vi "image_analysis_bkgndmagnetictrap.vi"(0 "2D Array In":i32[][](array[numeric]), 1 "File Path for \nbackground image":path=path "C:/data/MOT/08.05.02/metapictemp600c1v40a35msh100usd1.000motp0back.bmp", 2 "Ions or Neutral Atoms?":bool=TRUE, 3 "Delta_x (m)":dbl=2.33e-05 format="%.2e", 4 "Delta_y (m)":dbl=4.63e-05 format="%.2e", 5 "camera background with no image beam\nIt will be subtracted before the log is taken":i8=15, 6 "coilcurrent":dbl=40.0 format="%.2f", 7 "take new\nnew image":bool=TRUE, 8 "ROI Controls":T1, 10 "Image beam \nDetuning (MHz)":dbl=12.5 format="%.2f", 11 "Cut image?":bool, 12 "timeout(min 100ms)":u32=1000) -> (9 "Intensity Graph \natoms":sgl[][](graph), 13 "Intensity Graph \nbackground":sgl[][](graph), 14 "X  side":cluster{cluster{dbl, dbl}[]}[](graph)=[{[{0.0, -0.00023040071411132814}, {2.33e-05, -0.00023119197387695312}, {4.66e-05, -0.0002076152587890625}, {6.99e-05, -0.00020104497680664061}, {9.32e-05, -0.000178349951171875}, {0.0001165, -0.00020604686889648437}, {0.0001398, -0.00019964896850585938}, {0.0001631, -0.0001973317077636719}, {0.0001864, -0.00018958018798828126}, {0.0002097, -0.00018725162353515625}, {0.000233, -0.00018564649658203125}, {0.0002563, -0.0001972638854980469}, {0.0002796, -0.00018755399780273437}, {0.0003029, -0.00017615420532226563}, {0.0003262, -0.00017684373168945313}, {0.0003495, -0.00017816343994140626}, {0.0003728, -0.00018060221557617188}, {0.00039610000000000003, -0.00018643775634765626}, {0.0004194, -0.00021354122924804688}, {0.0004427, -0.00018863067626953125}, {0.000466, -0.00018703402709960938}, {0.0004893, -0.00018847242431640625}, {0.0005126, -0.00015889909057617189}, {0.0005359, -0.0001712625244140625}, {0.0005592, -0.00017300894775390625}, {0.0005825, -0.00016774424438476562}, {0.0006058, -0.00018329815063476563}, {0.0006291000000000001, -0.00014636327514648437}, {0.0006524, -0.00013831785888671874}, {0.0006757, -0.00016184935913085937}, {0.000699, -0.000178485595703125}, {0.0007223, -0.0001590545166015625}, {0.0007456, -0.00015677681884765626}, {0.0007689, -0.00013077545776367188}, {0.0007922000000000001, -0.00016876723022460937}, {0.0008155, -0.000126985888671875}, {0.0008388, -0.00016878983764648437}, {0.0008621, -0.00014658369750976562}, {0.0008854, -0.00016071333618164062}, {0.0009087, -0.00014554093017578125}, {0.000932, -0.00013422308959960938}, {0.0009553000000000001, -0.0001502178405761719}, {0.0009786, -0.00015147537841796876}, {0.0010019, -0.00014486270751953124}, {0.0010252, -0.00015495974731445314}, {0.0010485, -0.00012384345703125}, {0.0010718, -0.00012299850463867186}, {0.0010951000000000001, -0.00013838568115234374}, {0.0011184, -0.00016345731201171875}, {0.0011417, -0.0001566948669433594}, {0.001165, -0.00014931636962890626}, {0.0011883, -0.00010717896118164062}, {0.0012116, -0.00010879256591796875}, {0.0012349, -0.0001059722900390625}, {0.0012582000000000001, -0.0001241938720703125}, {0.0012815, -0.00013572083129882812}, {0.0013048, -0.00012067559204101562}, {0.0013281, -0.00012900077514648437}, {0.0013514, -9.90544189453125e-05}, {0.0013747, -0.0001157160888671875}, {0.001398, -0.00011736077880859375}, {0.0014213000000000001, -8.70498779296875e-05}, {0.0014446, -0.000123526953125}, {0.0014679, -0.0001004560791015625}, {0.0014912, -5.974576416015625e-05}, {0.0015145, -7.730042724609375e-05}, {0.0015378, -9.181156616210937e-05}, {0.0015611, -0.0001171064453125}, {0.0015844000000000001, -7.690197143554687e-05}, {0.0016077, -7.38019287109375e-05}, {0.001631, -9.62510986328125e-05}, {0.0016543, -4.338646850585937e-05}, {0.0016776, -9.5878076171875e-05}, {0.0017009, -7.96346435546875e-05}, {0.0017242, -7.93181396484375e-05}, {0.0017475000000000001, -6.642060546875e-05}, {0.0017708, -5.844301147460938e-05}, {0.0017941, -2.755279541015625e-05}, {0.0018174, -2.5744201660156252e-05}, {0.0018407, -5.0640625e-05}, {0.001864, -4.254151611328125e-05}, {0.0018873, -3.9766455078125e-05}, {0.0019106000000000001, -1.7760955810546876e-05}, {0.0019339000000000001, -2.0016046142578124e-05}, {0.0019572, -1.730032958984375e-05}, {0.0019805, 4.25584716796875e-06}, {0.0020038, -1.5260009765625e-06}, {0.0020271, 1.6353643798828126e-05}, {0.0020504, 4.45931396484375e-06}, {0.0020737, 1.56782470703125e-05}, {0.002097, 1.87754638671875e-05}, {0.0021203, 6.5250671386718754e-06}, {0.0021436, -7.1778564453125e-07}, {0.0021669000000000002, 2.6719146728515625e-05}, {0.0021902000000000002, 4.67182373046875e-05}, {0.0022135, 4.4092950439453123e-05}, {0.0022368, 5.912688598632813e-05}, {0.0022601, 6.413160400390626e-05}, {0.0022834, 5.6900054931640624e-05}, {0.0023067, 6.803703613281251e-05}, {0.00233, 8.644512939453125e-05}, {0.0023533, 7.566138916015625e-05}, {0.0023766, 6.502459716796875e-05}, {0.0023999, 8.933887939453125e-05}, {0.0024232, 9.000579833984375e-05}, {0.0024465, 0.0001182481201171875}, {0.0024698, 0.0001048871337890625}, {0.0024931000000000003, 0.0001308856689453125}, {0.0025164000000000002, 0.00013674946899414062}, {0.0025397, 0.0001610552734375}, {0.002563, 0.00014260196533203126}, {0.0025863, 0.0001531341979980469}, {0.0026096, 0.0001802150634765625}, {0.0026329, 0.00019327367553710937}, {0.0026562, 0.00022464429931640624}, {0.0026795, 0.000221123193359375}, {0.0027028, 0.00019760864868164063}, {0.0027261, 0.00019808905639648439}, {0.0027494, 0.00023230821533203126}, {0.0027727, 0.0002467458801269531}, {0.002796, 0.00025002678222656253}, {0.0028193000000000003, 0.00026431184692382814}, {0.0028426000000000002, 0.0002459941833496094}, {0.0028659000000000002, 0.00026929395751953126}, {0.0028892, 0.0003082606750488281}, {0.0029125, 0.0002984066650390625}, {0.0029358, 0.00030499107666015626}, {0.0029591, 0.00033020400390625}, {0.0029824, 0.0003341263916015625}, {0.0030057, 0.00035323531494140626}, {0.003029, 0.00035600755004882814}, {0.0030523, 0.00037995446166992186}, {0.0030756, 0.0003714258117675781}, {0.0030989, 0.0003785414978027344}, {0.0031222, 0.00038694580688476563}, {0.0031455, 0.0004150440063476563}, {0.0031688000000000003, 0.0004460359558105469}, {0.0031921000000000002, 0.0004576816040039063}, {0.0032154, 0.0004373829650878906}, {0.0032387, 0.00044043496704101564}, {0.003262, 0.00046968614501953124}, {0.0032853, 0.00046797928466796876}, {0.0033086, 0.0005343603271484375}, {0.0033319, 0.000518049072265625}, {0.0033552, 0.0005307911804199219}, {0.0033785, 0.0005506433227539062}, {0.0034018, 0.0005478513061523437}, {0.0034251, 0.0005569762268066407}, {0.0034484, 0.0005951799438476562}, {0.0034717, 0.0006168124206542969}, {0.0034950000000000003, 0.0006063564880371094}, {0.0035183000000000002, 0.0006301931884765625}, {0.0035416, 0.0006353505065917969}, {0.0035649, 0.0006507065979003907}, {0.0035882, 0.0006587463623046875}, {0.0036115, 0.0007066260559082031}, {0.0036348, 0.0006745715576171876}, {0.0036581, 0.0007187690673828125}, {0.0036814, 0.0007195122863769531}, {0.0037047, 0.0007214169616699219}, {0.003728, 0.0007334469360351563}, {0.0037513, 0.0007567438842773438}, {0.0037746, 0.0007910478210449218}, {0.0037979, 0.0007963803466796875}, {0.0038212000000000003, 0.0007861307067871094}, {0.0038445000000000003, 0.0008184621459960937}, {0.0038678000000000002, 0.0008249674316406251}, {0.0038911, 0.0008380316955566406}, {0.0039144, 0.0008839106323242187}, {0.0039377, 0.0008829582946777343}, {0.003961, 0.0009055233276367187}, {0.0039843000000000005, 0.0009045681640625}, {0.0040076, 0.0009299393432617188}, {0.0040309000000000005, 0.0009854631713867188}, {0.0040542, 0.0009813542724609375}, {0.0040775, 0.0009880488952636718}, {0.0041008, 0.001000581884765625}, {0.0041241, 0.0010300223999023437}, {0.0041474, 0.001029171795654297}, {0.0041707, 0.0010493347900390625}, {0.004194, 0.0010845712829589845}, {0.0042173, 0.0010739486206054688}, {0.0042406, 0.001092376495361328}, {0.0042639, 0.0011004558227539062}, {0.0042872, 0.0011284014221191407}, {0.0043105, 0.0011756170227050782}, {0.0043338000000000005, 0.001184140020751953}, {0.0043571, 0.0011864940185546875}, {0.0043804000000000004, 0.0012101272521972655}, {0.0044037, 0.001194449005126953}, {0.004427, 0.0012500717407226563}, {0.0044503, 0.0012585269165039062}, {0.0044736, 0.0012805493713378907}, {0.0044969, 0.0012812869384765625}, {0.0045202, 0.0012850680297851562}, {0.0045435, 0.001292859112548828}, {0.0045668, 0.0013328488159179688}, {0.0045901, 0.0013298702880859374}, {0.0046134, 0.0013652791625976563}, {0.0046367, 0.001366519744873047}, {0.00466, 0.0013854901977539062}, {0.0046833000000000005, 0.0014075380859375}, {0.0047066, 0.0014307163452148438}, {0.0047299, 0.001454810205078125}, {0.0047532, 0.0014336440063476563}, {0.0047765, 0.0014266159240722655}, {0.0047998, 0.0014909622985839843}, {0.0048231, 0.0014609170349121094}, {0.0048464, 0.0015016838684082032}, {0.0048697, 0.0015183624938964844}, {0.004893, 0.0015467969787597657}, {0.0049163, 0.0015608559692382813}, {0.0049396, 0.0015447057922363281}, {0.0049629, 0.0015464098266601562}, {0.0049862000000000005, 0.0015989127380371094}, {0.0050095, 0.001574869744873047}, {0.0050328000000000005, 0.00164387607421875}, {0.0050561, 0.001618668798828125}, {0.0050794, 0.0016376618591308594}, {0.0051027, 0.0016571861938476562}, {0.005126, 0.0016686396789550781}, {0.0051493, 0.0017015108703613282}, {0.0051726, 0.0016855048156738282}, {0.0051959, 0.001690854296875}, {0.0052192, 0.0017352072326660157}, {0.0052425, 0.001697243719482422}, {0.0052658, 0.001747906951904297}, {0.0052891, 0.0017650772888183593}, {0.0053124, 0.001771729522705078}, {0.0053357000000000005, 0.0017894961303710937}, {0.005359, 0.00176170595703125}, {0.0053823000000000005, 0.0017409551696777343}, {0.0054056, 0.0017913838500976562}, {0.0054289, 0.0017596119445800781}, {0.0054522, 0.0018210221801757812}, {0.0054755, 0.001803001239013672}, {0.0054988, 0.0018012209045410157}, {0.0055221, 0.0017957386047363281}, {0.0055454, 0.0017480991149902345}, {0.0055687, 0.0017993049255371095}, {0.005592, 0.0017956142639160156}, {0.0056153, 0.0017572579467773437}, {0.0056386000000000006, 0.0017667954528808594}, {0.0056619, 0.0017284334838867188}, {0.0056852000000000005, 0.0017505181091308595}, {0.0057085, 0.0017459655395507814}, {0.0057318000000000004, 0.0017314883117675781}, {0.0057551, 0.0017498059753417968}, {0.0057784, 0.0016802429382324219}, {0.0058017, 0.0016734070190429688}, {0.005825, 0.0017002109436035156}, {0.0058483, 0.0016686877197265625}, {0.0058716, 0.0016841088073730468}, {0.0058949, 0.0016317697998046875}, {0.0059182, 0.0016261857666015624}, {0.0059415, 0.0016222972900390626}, {0.0059648, 0.0015984068969726562}, {0.0059881000000000005, 0.0015912149108886719}, {0.0060114, 0.0015728605102539063}, {0.0060347000000000005, 0.0015469467529296876}, {0.006058, 0.001551163037109375}, {0.0060813, 0.00149213505859375}, {0.0061046, 0.0015037891845703125}, {0.0061279, 0.001491109246826172}, {0.0061512, 0.001486989044189453}, {0.0061745, 0.0014903462463378907}, {0.0061978, 0.0014408331665039062}, {0.0062211, 0.0014393523803710939}, {0.0062444, 0.001456573583984375}, {0.0062677, 0.0014138681640625001}, {0.006291, 0.0014108783325195312}, {0.0063143, 0.0013740904052734375}, {0.0063376000000000005, 0.0013829835998535156}, {0.0063609, 0.0013793635864257812}, {0.0063842000000000005, 0.0013252555480957032}, {0.0064075, 0.0013514603759765625}, {0.0064308, 0.001354628240966797}, {0.0064541, 0.0013122393249511719}, {0.0064774, 0.0013079213073730468}, {0.0065007, 0.0012758922424316406}, {0.006524, 0.001295345928955078}, {0.0065473, 0.001262678204345703}, {0.0065706, 0.0012528157165527345}, {0.0065939, 0.00124372470703125}, {0.0066172, 0.0012110513305664062}, {0.006640500000000001, 0.0012050151489257812}, {0.0066638, 0.0012236351867675782}, {0.0066871000000000005, 0.0012089064514160157}, {0.0067104, 0.0012079032470703125}, {0.0067337000000000004, 0.0011969132141113282}, {0.006757, 0.0011709938049316406}, {0.0067803, 0.001169188037109375}, {0.0068036, 0.0011361529418945312}, {0.0068269, 0.0011614676025390625}, {0.0068502, 0.0011093857543945313}, {0.0068735, 0.001095261767578125}, {0.0068968, 0.0010902287902832032}, {0.0069201, 0.0010482552856445314}, {0.0069434, 0.0010696192993164062}, {0.0069667, 0.0010469384033203126}, {0.0069900000000000006, 0.0010472775146484375}, {0.0070133, 0.0010401024841308593}, {0.0070366000000000005, 0.0010032099975585938}, {0.0070599, 0.001027213427734375}, {0.0070832, 0.0010276994873046875}, {0.0071065, 0.0010024526489257812}, {0.0071298, 0.0009888966735839843}, {0.0071531, 0.00094928564453125}, {0.0071764, 0.0009297923950195312}, {0.0071997, 0.0009235018798828125}, {0.007223, 0.0009235923095703125}, {0.0072463, 0.0009299223876953125}, {0.0072696, 0.0009213570007324219}, {0.007292900000000001, 0.0008789002624511719}, {0.0073162, 0.0009023413330078125}, {0.0073395000000000005, 0.0008445200256347657}, {0.0073628, 0.00087694189453125}, {0.0073861000000000005, 0.0008312777282714844}, {0.0074094, 0.0008174109008789063}, {0.0074327, 0.0007991554077148437}, {0.007456, 0.0007847120910644531}, {0.0074793, 0.0007734451171875}, {0.0075026, 0.0007596206787109375}, {0.0075259, 0.0007575690551757813}, {0.0075492, 0.0007569049621582031}, {0.0075725, 0.0007450445434570313}, {0.0075958, 0.0007419247192382813}, {0.0076191, 0.0007280974548339844}, {0.007642400000000001, 0.0007225501586914062}, {0.0076657, 0.0007196733642578125}, {0.0076890000000000005, 0.0006959101379394532}, {0.0077123, 0.0006711521850585937}, {0.0077356000000000005, 0.0006568077758789063}, {0.0077589, 0.0006257084411621093}, {0.0077822, 0.0006641862731933594}, {0.0078055, 0.0006440458862304688}, {0.0078288, 0.0005976017639160156}, {0.0078521, 0.0005779502624511718}, {0.0078754, 0.000566338525390625}, {0.0078987, 0.0005991984130859375}, {0.007922, 0.000589217236328125}, {0.0079453, 0.0005806659790039062}, {0.007968600000000001, 0.0005688451232910156}, {0.0079919, 0.0005396080749511719}, {0.0080152, 0.0005325545593261718}, {0.0080385, 0.0005257525512695312}, {0.008061800000000001, 0.0005257695068359375}, {0.0080851, 0.0005317604736328125}, {0.0081084, 0.0005006583129882813}, {0.0081317, 0.0004965296325683593}, {0.008155, 0.00046909835205078125}, {0.0081783, 0.0004614259582519531}, {0.0082016, 0.00047987361450195314}, {0.0082249, 0.00047146365356445314}, {0.0082482, 0.0004377051208496094}, {0.0082715, 0.00043660300903320315}, {0.0082948, 0.00042543494262695314}, {0.0083181, 0.00040906151733398436}, {0.0083414, 0.000402072998046875}, {0.008364700000000001, 0.00041385711669921876}, {0.008388, 0.00040132130126953124}, {0.0084113, 0.0003789427795410156}, {0.0084346, 0.0003775580749511719}, {0.0084579, 0.00038707862548828124}, {0.0084812, 0.00038257409667968753}, {0.0085045, 0.0003654150634765625}, {0.0085278, 0.0003459642028808594}, {0.0085511, 0.0003380883422851563}, {0.0085744, 0.0003251879821777344}, {0.0085977, 0.0003157691650390625}, {0.008621, 0.00032381175537109377}, {0.0086443, 0.0003224129211425781}, {0.008667600000000001, 0.00025898214721679685}, {0.0086909, 0.00028225648803710936}, {0.0087142, 0.00029155944213867186}, {0.0087375, 0.0002851587158203125}, {0.008760800000000001, 0.0002583830505371094}, {0.0087841, 0.000267852734375}, {0.0088074, 0.00026862703857421876}, {0.0088307, 0.0002457794128417969}, {0.008854, 0.00026741754150390627}, {0.0088773, 0.00025229600219726564}, {0.0089006, 0.0002459094055175781}, {0.0089239, 0.00023786964111328126}, {0.0089472, 0.0001981879638671875}, {0.008970500000000001, 0.000217008642578125}, {0.0089938, 0.0001958396179199219}, {0.0090171, 0.00017722805786132812}, {0.0090404, 0.000195870703125}, {0.009063700000000001, 0.00019522356567382813}, {0.009087, 0.00017875971069335937}, {0.0091103, 0.00014470445556640624}, {0.0091336, 0.00015979773559570313}, {0.0091569, 0.00017249180297851561}, {0.0091802, 0.00016237498168945313}, {0.0092035, 0.00013187756958007811}, {0.0092268, 0.00015409783935546874}, {0.0092501, 0.00013750681762695312}, {0.0092734, 0.00011370968017578125}, {0.0092967, 0.00013704901733398438}, {0.00932, 0.0001348645751953125}, {0.0093433, 0.00012259439697265626}, {0.009366600000000001, 0.00010125016479492187}, {0.0093899, 0.00010383871459960938}, {0.0094132, 0.00011125394897460937}, {0.0094365, 9.88509521484375e-05}, {0.0094598, 0.00010897625122070313}, {0.0094831, 8.164387817382812e-05}, {0.0095064, 7.74982421875e-05}, {0.0095297, 7.682001953125e-05}, {0.009553, 6.663820190429688e-05}, {0.0095763, 7.056624145507813e-05}, {0.0095996, 7.633113403320313e-05}, {0.0096229, 7.789104614257812e-05}, {0.0096462, 4.640738525390625e-05}, {0.009669500000000001, 4.845053100585938e-05}, {0.0096928, 4.96458984375e-05}, {0.0097161, 5.6210528564453123e-05}, {0.0097394, 4.7902301025390626e-05}, {0.009762700000000001, 5.1163421630859375e-05}, {0.009786, 1.9948223876953125e-05}, {0.0098093, 1.3098175048828125e-05}, {0.0098326, 7.392626953125e-06}, {0.0098559, 2.1344232177734376e-05}, {0.0098792, 5.2904193115234375e-05}, {0.0099025, 2.7176947021484377e-05}, {0.0099258, 2.225135498046875e-05}, {0.0099491, 1.2999267578125e-07}, {0.009972400000000001, 3.179168701171875e-06}, {0.0099957, 2.6894354248046875e-05}, {0.010019, 1.855504150390625e-05}, {0.0100423, 6.3865966796875e-07}, {0.010065600000000001, -2.16126953125e-05}, {0.0100889, -3.361158447265625e-05}, {0.0101122, -2.79992919921875e-05}, {0.0101355, -3.770070190429687e-05}, {0.0101588, -3.201776123046875e-05}, {0.0101821, -1.386400146484375e-05}, {0.0102054, -5.105038452148438e-05}, {0.0102287, -4.5466351318359374e-05}, {0.010252, -6.17634765625e-05}, {0.010275300000000001, -5.5396661376953125e-05}, {0.0102986, -6.0681146240234377e-05}, {0.0103219, -3.617752685546875e-05}, {0.0103452, -6.318491821289062e-05}, {0.010368500000000001, -6.894981079101563e-05}, {0.0103918, -7.838558349609376e-05}, {0.0104151, -6.183695068359375e-05}, {0.0104384, -7.396583251953125e-05}, {0.0104617, -6.277798461914063e-05}, {0.010485, -8.242383422851562e-05}, {0.0105083, -0.00010097887573242188}, {0.0105316, -9.987393798828126e-05}, {0.0105549, -8.323770141601563e-05}, {0.0105782, -8.575842895507812e-05}, {0.0106015, -6.663537597656251e-05}, {0.0106248, -0.0001043445556640625}, {0.0106481, -0.00011336774291992187}, {0.010671400000000001, -0.00011448115844726562}, {0.0106947, -0.00010283833618164062}, {0.010718, -7.121620483398437e-05}, {0.0107413, -8.04485107421875e-05}, {0.010764600000000001, -8.028743286132812e-05}, {0.0107879, -9.259717407226563e-05}, {0.0108112, -9.686432495117187e-05}, {0.0108345, -8.311336059570312e-05}, {0.0108578, -9.37416748046875e-05}, {0.0108811, -0.00011418443603515625}, {0.0109044, -0.00013360421142578126}, {0.0109277, -0.00010200751342773437}, {0.010951, -0.00013351095581054688}, {0.010974300000000001, -0.00013001810913085938}, {0.0109976, -0.00011018574829101562}, {0.0110209, -0.000120701025390625}, {0.0110442, -0.0001419180908203125}, {0.011067500000000001, -0.00015386611328125}, {0.0110908, -0.00016053247680664063}, {0.0111141, -0.00013401397094726561}, {0.0111374, -0.00014181070556640624}, {0.0111607, -0.00014792883911132813}, {0.011184, -0.00014493052978515624}, {0.0112073, -0.00017492775268554688}, {0.0112306, -0.00016084898071289062}, {0.0112539, -0.00011132742309570313}, {0.011277200000000001, -0.00012937379760742188}, {0.0113005, -0.00013684555053710939}, {0.0113238, -0.0001691826416015625}, {0.0113471, -0.0001933499755859375}, {0.011370400000000001, -0.00015698876342773438}, {0.0113937, -0.00014668260498046875}, {0.011417, -0.00015133408203125}, {0.0114403, -0.000162954296875}, {0.011463600000000001, -0.00016880679321289063}, {0.0114869, -0.00018441156616210938}, {0.0115102, -0.0001858443115234375}, {0.0115335, -0.00015983164672851564}, {0.0115568, -0.00015530733642578126}, {0.0115801, -0.00017589421997070312}, {0.0116034, -0.00018566062622070312}, {0.0116267, -0.00016709428100585938}, {0.01165, -0.00019034036254882811}, {0.011673300000000001, -0.00016057486572265624}, {0.0116966, -0.0001708697204589844}, {0.0117199, -0.00015639531860351562}, {0.0117432, -0.0001735910888671875}, {0.011766500000000001, -0.00018023484497070312}, {0.0117898, -0.00017295525512695312}, {0.0118131, -0.00017341588134765624}, {0.0118364, -0.00016610238037109376}, {0.0118597, -0.00016709710693359376}, {0.011883, -0.00018562388916015625}, {0.0119063, -0.00019376538696289062}, {0.0119296, -0.00019743909301757811}, {0.0119529, -0.000188975439453125}, {0.011976200000000001, -0.000169171337890625}, {0.0119995, -0.0001794153259277344}, {0.0120228, -0.00019441817626953125}, {0.0120461, -0.00018920433959960937}, {0.012069400000000001, -0.00021696060180664064}, {0.0120927, -0.00020950863037109374}, {0.012116, -0.00019751256713867188}, {0.0121393, -0.00020696529541015625}, {0.0121626, -0.00022381065063476561}, {0.0121859, -0.00020375221557617187}, {0.0122092, -0.00020652727661132813}, {0.0122325, -0.00018872110595703125}, {0.0122558, -0.00016852985229492187}, {0.012279100000000001, -0.00017135012817382812}]}, {[{0.0, -0.00014104949248999906}, {2.33e-05, -0.00013981727171733847}, {4.66e-05, -0.00013856446463566041}, {6.99e-05, -0.0001372907360713168}, {9.32e-05, -0.00013599574566188237}, {0.0001165, -0.00013467914778464025}, {0.0001398, -0.00013334059148439962}, {0.0001631, -0.00013197972040065195}, {0.0001864, -0.00013059617269407412}, {0.0002097, -0.00012918958097238675}, {0.000233, -0.00012775957221557732}, {0.0002563, -0.0001263057677004986}, {0.0002796, -0.00012482778292485336}, {0.0003029, -0.0001233252275305777}, {0.0003262, -0.00012179770522663655}, {0.0003495, -0.00012024481371124538}, {0.0003728, -0.00011866614459353325}, {0.00039610000000000003, -0.00011706128331466457}, {0.0004194, -0.00011542980906843669}, {0.0004427, -0.00011377129472137248}, {0.000466, -0.00011208530673232863}, {0.0004893, -0.00011037140507164106}, {0.0005126, -0.00010862914313983072}, {0.0005359, -0.0001068580676858948}, {0.0005592, -0.00010505771872520905}, {0.0005825, -0.00010322762945707002}, {0.0006058, -0.00010136732618190591}, {0.0006291000000000001, -9.947632821818837e-05}, {0.0006524, -9.755414781907809e-05}, {0.0006757, -9.56002900888396e-05}, {0.000699, -9.361425289906293e-05}, {0.0007223, -9.15955268047311e-05}, {0.0007456, -8.954359496017582e-05}, {0.0007689, -8.745793303496495e-05}, {0.0007922000000000001, -8.533800912976849e-05}, {0.0008155, -8.318328369225223e-05}, {0.0008388, -8.099320943305044e-05}, {0.0008621, -7.876723124187247e-05}, {0.0008854, -7.650478610380028e-05}, {0.0009087, -7.42053030158376e-05}, {0.000932, -7.186820290377375e-05}, {0.0009553000000000001, -6.949289853942946e-05}, {0.0009786, -6.707879445835457e-05}, {0.0010019, -6.462528687805136e-05}, {0.0010252, -6.213176361680116e-05}, {0.0010485, -5.9597604013175534e-05}, {0.0010718, -5.702217884631736e-05}, {0.0010951000000000001, -5.440485025708157e-05}, {0.0011184, -5.17449716701296e-05}, {0.0011417, -4.9041887717075847e-05}, {0.001165, -4.629493416078989e-05}, {0.0011883, -4.3503437820962705e-05}, {0.0012116, -4.0666716501050344e-05}, {0.0012349, -3.778407891671416e-05}, {0.0012582000000000001, -3.485482462588216e-05}, {0.0012815, -3.18782439605621e-05}, {0.0013048, -2.8853617960542617e-05}, {0.0013281, -2.5780218309125948e-05}, {0.0013514, -2.2657307271041507e-05}, {0.0013747, -1.9484137632697125e-05}, {0.001398, -1.6259952644931817e-05}, {0.0014213000000000001, -1.2983985968441451e-05}, {0.0014446, -9.65546162205678e-06}, {0.0014679, -6.273593934060806e-06}, {0.0014912, -2.837587496742161e-06}, {0.0015145, 6.533628756111433e-07}, {0.0015378, 4.200072185063217e-06}, {0.0015611, 7.803365284503273e-06}, {0.0015844000000000001, 1.1464076908006274e-05}, {0.0016077, 1.5183051696836682e-05}, {0.001631, 1.8961144220840576e-05}, {0.0016543, 2.2799218994958835e-05}, {0.0016776, 2.6698150490583402e-05}, {0.0017009, 3.0658823141465644e-05}, {0.0017242, 3.4682131343873173e-05}, {0.0017475000000000001, 3.87689794506781e-05}, {0.0017708, 4.2920281759045554e-05}, {0.0017941, 4.713696249137747e-05}, {0.0018174, 5.141995576915033e-05}, {0.0018407, 5.577020557927103e-05}, {0.001864, 6.018866573255787e-05}, {0.0018873, 6.467629981393693e-05}, {0.0019106000000000001, 6.923408112392624e-05}, {0.0019339000000000001, 7.386299261096143e-05}, {0.0019572, 7.85640267940981e-05}, {0.0019805, 8.333818567560471e-05}, {0.0020038, 8.818648064294049e-05}, {0.0020271, 9.310993235958977e-05}, {0.0020504, 9.810957064420282e-05}, {0.0020737, 0.0001031864343374686}, {0.002097, 0.0001083415711561212}, {0.0021203, 0.00011357603753345596}, {0.0021436, 0.00011889089844570489}, {0.0021669000000000002, 0.0001242872272235936}, {0.0021902000000000002, 0.0001297661053483724}, {0.0022135, 0.00013532862223158732}, {0.0022368, 0.00014097587497782102}, {0.0022601, 0.0001467089681296067}, {0.0022834, 0.000152529013393681}, {0.0023067, 0.0001584371293477089}, {0.00233, 0.0001644344411265769}, {0.0023533, 0.00017052208008731386}, {0.0023766, 0.00017670118345165982}, {0.0023999, 0.00018297289392526202}, {0.0024232, 0.00018933835929243721}, {0.0024465, 0.000195798731985394}, {0.0024698, 0.0002023551686267653}, {0.0024931000000000003, 0.0002090088295442538}, {0.0025164000000000002, 0.00021576087825614384}, {0.0025397, 0.00022261248092638687}, {0.002563, 0.00022956480578790905}, {0.0025863, 0.00023661902253274285}, {0.0026096, 0.00024377630166752401}, {0.0026329, 0.00025103781383284}, {0.0026562, 0.00025840472908485586}, {0.0026795, 0.00026587821613758194}, {0.0027028, 0.0002734594415640851}, {0.0027261, 0.00028114956895487834}, {0.0027494, 0.0002889497580316582}, {0.0027727, 0.00029686116371448743}, {0.002796, 0.00030488493514045086}, {0.0028193000000000003, 0.00031302221463173777}, {0.0028426000000000002, 0.00032127413661102764}, {0.0028659000000000002, 0.00032964182646198173}, {0.0028892, 0.00033812639933255775}, {0.0029125, 0.00034672895887878863}, {0.0029358, 0.00035545059594658}, {0.0029591, 0.0003642923871889965}, {0.0029824, 0.0003732553936164198}, {0.0030057, 0.0003823406590768732}, {0.003029, 0.00039154920866371715}, {0.0030523, 0.00040088204704782893}, {0.0030756, 0.00041034015673128803}, {0.0030989, 0.0004199244962194943}, {0.0031222, 0.00042963599810855375}, {0.0031455, 0.00043947556708467207}, {0.0031688000000000003, 0.00044944407783220164}, {0.0031921000000000002, 0.00045954237284689486}, {0.0032154, 0.0004697712601508261}, {0.0032387, 0.00048013151090534756}, {0.003262, 0.0004906238569183633}, {0.0032853, 0.0005012489880421125}, {0.0033086, 0.000512007549457573}, {0.0033319, 0.0005229001388415179}, {0.0033552, 0.0005339273034121817}, {0.0033785, 0.0005450895368494259}, {0.0034018, 0.0005563872760852344}, {0.0034251, 0.0005678208979603144}, {0.0034484, 0.0005793907157425372}, {0.0034717, 0.0005910969755029226}, {0.0034950000000000003, 0.0006029398523448503}, {0.0035183000000000002, 0.0006149194464821778}, {0.0035416, 0.0006270357791619623}, {0.0035649, 0.0006392887884275047}, {0.0035882, 0.0006516783247174985}, {0.0036115, 0.0006642041462971361}, {0.0036348, 0.0006768659145171294}, {0.0036581, 0.0006896631888967342}, {0.0036814, 0.000702595422027037}, {0.0037047, 0.0007156619542909608}, {0.003728, 0.0007288620083966925}, {0.0037513, 0.0007421946837215215}, {0.0037746, 0.000755658950463419}, {0.0037979, 0.0007692536435980739}, {0.0038212000000000003, 0.0007829774566395585}, {0.0038445000000000003, 0.0007968289352033078}, {0.0038678000000000002, 0.0008108064703706903}, {0.0038911, 0.0008249082918551056}, {0.0039144, 0.0008391324609702966}, {0.0039377, 0.0008534768634024065}, {0.003961, 0.0008679392017882457}, {0.0039843000000000005, 0.0008825169881032757}, {0.0040076, 0.0008972075358639875}, {0.0040309000000000005, 0.0009120079521506221}, {0.0040542, 0.0009269151294575935}, {0.0040775, 0.0009419257373805432}, {0.0041008, 0.0009570362141506277}, {0.0041241, 0.0009722427580285325}, {0.0041474, 0.0009875413185726916}, {0.0041707, 0.0010029275877984267}, {0.004194, 0.0010183969912470597}, {0.0042173, 0.001033944678986653}, {0.0042406, 0.0010495655165687584}, {0.0042639, 0.0010652540759685447}, {0.0042872, 0.0010810046265387978}, {0.0043105, 0.0010968111260116899}, {0.0043338000000000005, 0.001112667211585733}, {0.0043571, 0.0011285661911391315}, {0.0043804000000000004, 0.0011445010346146738}, {0.0044037, 0.0011604643656254344}, {0.004427, 0.0011764484533348654}, {0.0044503, 0.0011924452046692612}, {0.0044736, 0.0012084461569251562}, {0.0044969, 0.0012244424708388088}, {0.0045202, 0.0012404249241896204}, {0.0045435, 0.0012563839060139549}, {0.0045668, 0.0012723094115104313}, {0.0045901, 0.0012881910377221634}, {0.0046134, 0.0013040179800856493}, {0.0046367, 0.001319779029939868}, {0.00466, 0.0013354625730926113}, {0.0046833000000000005, 0.0013510565895439343}, {0.0047066, 0.0013665486544688257}, {0.0047299, 0.0013819259405625018}, {0.0047532, 0.0013971752218520192}, {0.0047765, 0.0014122828790769724}, {0.0047998, 0.0014272349067396058}, {0.0048231, 0.001442016921920603}, {0.0048464, 0.0014566141749506997}, {0.0048697, 0.0014710115620199507}, {0.004893, 0.001485193639795481}, {0.0049163, 0.001499144642104625}, {0.0049396, 0.0015128484987229252}, {0.0049629, 0.0015262888562851747}, {0.0049862000000000005, 0.0015394491013117591}, {0.0050095, 0.001552312385311449}, {0.0050328000000000005, 0.0015648616518844068}, {0.0050561, 0.0015770796657044667}, {0.0050794, 0.0015889490432060942}, {0.0051027, 0.0016004522847367188}, {0.005126, 0.001611571807856486}, {0.0051493, 0.0016222899813706356}, {0.0051726, 0.0016325891595587387}, {0.0051959, 0.0016424517159108558}, {0.0052192, 0.00165186007547991}, {0.0052425, 0.0016607967446911841}, {0.0052658, 0.001669244337081019}, {0.0052891, 0.0016771855929139455}, {0.0053124, 0.001684603389861558}, {0.0053357000000000005, 0.001691480740763498}, {0.005359, 0.001697800772654961}, {0.0053823000000000005, 0.0017035466782173198}, {0.0054056, 0.0017087016255587506}, {0.0054289, 0.0017132486025734628}, {0.0054522, 0.0017171701530177502}, {0.0054755, 0.0017204479199437559}, {0.0054988, 0.0017230618100190975}, {0.0055221, 0.0017249882910849862}, {0.0055454, 0.0017261961360618139}, {0.0055687, 0.0017266273137008913}, {0.005592, 0.0017261737297977326}, {0.0056153, 0.0017249462798169639}, {0.0056386000000000006, 0.0017230012013243398}, {0.0056619, 0.0017203694086035948}, {0.0056852000000000005, 0.001717074306146829}, {0.0057085, 0.0017131359248754889}, {0.0057318000000000004, 0.0017085725893547189}, {0.0057551, 0.0017034017392668734}, {0.0057784, 0.0016976403791361065}, {0.0058017, 0.0016913053385510994}, {0.005825, 0.0016844134256319818}, {0.0058483, 0.0016769815158938254}, {0.0058716, 0.00166902659991218}, {0.0058949, 0.0016605658037011286}, {0.0059182, 0.0016516163905444321}, {0.0059415, 0.001642195750034317}, {0.0059648, 0.001632321378259561}, {0.0059881000000000005, 0.0016220108519350081}, {0.0060114, 0.0016112817985067481}, {0.0060347000000000005, 0.0016001518637494172}, {0.006058, 0.0015886386780064564}, {0.0060813, 0.001576759821957957}, {0.0061046, 0.0015645327926014033}, {0.0061279, 0.0015519749699774883}, {0.0061512, 0.0015391035850529492}, {0.0061745, 0.0015259356890760711}, {0.0061978, 0.0015124881246422906}, {0.0062211, 0.0014987774986429231}, {0.0062444, 0.001484820157216683}, {0.0062677, 0.0014706321627791215}, {0.006291, 0.0014562292731679662}, {0.0063143, 0.0014416269229113134}, {0.0063376000000000005, 0.0014268402065999105}, {0.0063609, 0.001411883864323507}, {0.0063842000000000005, 0.001396772269113986}, {0.0064075, 0.0013815194163241055}, {0.0064308, 0.0013661389148597654}, {0.0064541, 0.0013506439801754691}, {0.0064774, 0.0013350474289365798}, {0.0065007, 0.0013193616752479591}, {0.006524, 0.0013035987283461761}, {0.0065473, 0.0012877701916515958}, {0.0065706, 0.0012718872630769402}, {0.0065939, 0.0012559607364903047}, {0.0066172, 0.0012400010042327764}, {0.006640500000000001, 0.0012240180605937448}, {0.0066638, 0.0012080215061504188}, {0.0066871000000000005, 0.0011920205528819733}, {0.0067104, 0.001176024029972957}, {0.0067337000000000004, 0.0011600403902250105}, {0.006757, 0.0011440777170005547}, {0.0067803, 0.0011281437316267215}, {0.0068036, 0.0011122458011924986}, {0.0068269, 0.0010963909466766484}, {0.0068502, 0.0010805858513485412}, {0.0068735, 0.0010648368693884293}, {0.0068968, 0.0010491500346780237}, {0.0069201, 0.0010335310697163042}, {0.0069434, 0.0010179853946194987}, {0.0069667, 0.001002518136167861}, {0.0069900000000000006, 0.000987134136865492}, {0.0070133, 0.0009718379639827566}, {0.0070366000000000005, 0.0009566339185540345}, {0.0070599, 0.0009415260443064846}, {0.0070832, 0.0009265181364982474}, {0.0071065, 0.0009116137506470912}, {0.0071298, 0.0008968162111328542}, {0.0071531, 0.0008821286196592547}, {0.0071764, 0.0008675538635626299}, {0.0071997, 0.000853094623957049}, {0.007223, 0.00083875338370691}, {0.0072463, 0.0008245324352197122}, {0.0072696, 0.00081043388805307}, {0.007292900000000001, 0.0007964596763313487}, {0.0073162, 0.0007826115659684244}, {0.0073395000000000005, 0.0007688911616941364}, {0.0073628, 0.0007552999138829309}, {0.0073861000000000005, 0.0007418391251840176}, {0.0074094, 0.0007285099569531342}, {0.0074327, 0.0007153134354866465}, {0.007456, 0.0007022504580593267}, {0.0074793, 0.000689321798767637}, {0.0075026, 0.0006765281141808267}, {0.0075259, 0.0006638699488025085}, {0.0075492, 0.0006513477403457485}, {0.0075725, 0.0006389618248249593}, {0.0075958, 0.0006267124414681583}, {0.0076191, 0.0006145997374533254}, {0.007642400000000001, 0.0006026237724727872}, {0.0076657, 0.0005907845231296635}, {0.0076890000000000005, 0.0005790818871705275}, {0.0077123, 0.0005675156875585096}, {0.0077356000000000005, 0.0005560856763911087}, {0.0077589, 0.0005447915386670336}, {0.0077822, 0.0005336328959063783}, {0.0078055, 0.0005226093096284628}, {0.0078288, 0.0005117202846916198}, {0.0078521, 0.0005009652724992067}, {0.0078754, 0.0004903436740760549}, {0.0078987, 0.00047985484301952565}, {0.007922, 0.0004694980883292926}, {0.0079453, 0.00045927267711987465}, {0.007968600000000001, 0.00044917783721989756}, {0.0079919, 0.0004392127596619677}, {0.0080152, 0.00042937660106695806}, {0.0080385, 0.0004196684859264361}, {0.008061800000000001, 0.000410087508786845}, {0.0080851, 0.0004006327363389904}, {0.0081084, 0.0003913032094162652}, {0.0081317, 0.00038209794490497807}, {0.008155, 0.0003730159375700266}, {0.0081783, 0.0003640561617990912}, {0.0082016, 0.00035521757326841013}, {0.0082249, 0.0003464991105331239}, {0.0082482, 0.00033789969654505835}, {0.0082715, 0.0003294182401007523}, {0.0082948, 0.0003210536372224228}, {0.0083181, 0.0003128047724744942}, {0.0083414, 0.00030467052021820596}, {0.008364700000000001, 0.00029664974580674976}, {0.008388, 0.0002887413067232942}, {0.0084113, 0.0002809440536641687}, {0.0084346, 0.00027325683156941607}, {0.0084579, 0.00026567848060282006}, {0.0084812, 0.0002582078370834628}, {0.0085045, 0.00025084373437077637}, {0.0085278, 0.00024358500370499618}, {0.0085511, 0.00023643047500483572}, {0.0085744, 0.00022937897762415348}, {0.0085977, 0.000222429341069303}, {0.008621, 0.00021558039567880826}, {0.0086443, 0.00020883097326692586}, {0.008667600000000001, 0.00020217990773261523}, {0.0086909, 0.00019562603563536948}, {0.0087142, 0.0001891681967393044}, {0.0087375, 0.000182805234526859}, {0.008760800000000001, 0.00017653599668339233}, {0.0087841, 0.0001703593355539283}, {0.0088074, 0.00016427410857323903}, {0.0088307, 0.00015827917867042288}, {0.008854, 0.0001523734146490724}, {0.0088773, 0.00014655569154410048}, {0.0089006, 0.00014082489095623796}, {0.0089239, 0.00013517990136518884}, {0.0089472, 0.00012961961842237378}, {0.008970500000000001, 0.00012414294522417128}, {0.0089938, 0.00011874879256652075}, {0.0090171, 0.00011343607918171719}, {0.0090404, 0.000108203731958202}, {0.009063700000000001, 0.00010305068614410835}, {0.009087, 9.797588553530289e-05}, {0.0091103, 9.29782826486249e-05}, {0.0091336, 8.805683888100608e-05}, {0.0091569, 8.321052465511323e-05}, {0.0091802, 7.84383195521429e-05}, {0.0092035, 7.373921243236161e-05}, {0.0092268, 6.91122015439708e-05}, {0.0092501, 6.45562946208391e-05}, {0.0092734, 6.007050896963525e-05}, {0.0092967, 5.5653871546863024e-05}, {0.00932, 5.130541902628843e-05}, {0.0093433, 4.702419785721733e-05}, {0.009366600000000001, 4.28092643140741e-05}, {0.0093899, 3.865968453770673e-05}, {0.0094132, 3.457453456882615e-05}, {0.0094365, 3.0552900373976854e-05}, {0.0094598, 2.659387786440848e-05}, {0.0094831, 2.269657290821349e-05}, {0.0095064, 1.886010133607251e-05}, {0.0095297, 1.50835889409426e-05}, {0.009553, 1.1366171471999242e-05}, {0.0095763, 7.706994623140118e-06}, {0.0095996, 4.105214016337679e-06}, {0.0096229, 5.599951801230719e-07}, {0.0096462, -2.9294864765377238e-06}, {0.009669500000000001, -6.36404569471648e-06}, {0.0096928, -9.74448740010137e-06}, {0.0097161, -1.3071606741449315e-05}, {0.0097394, -1.6346189132684726e-05}, {0.009762700000000001, -1.9569010298435754e-05}, {0.009786, -2.2740836322799407e-05}, {0.0098093, -2.5862423701142663e-05}, {0.0098326, -2.893451939474859e-05}, {0.0098559, -3.195786088813309e-05}, {0.0098792, -3.493317624885732e-05}, {0.0099025, -3.7861184189674853e-05}, {0.0099258, -4.074259413285356e-05}, {0.0099491, -4.357810627652714e-05}, {0.009972400000000001, -4.636841166293011e-05}, {0.0099957, -4.911419224838096e-05}, {0.010019, -5.1816120974883993e-05}, {0.0100423, -5.447486184322249e-05}, {0.010065600000000001, -5.709106998742835e-05}, {0.0100889, -5.9665391750511546e-05}, {0.0101122, -6.219846476134356e-05}, {0.0101355, -6.46909180125884e-05}, {0.0101588, -6.714337193958672e-05}, {0.0101821, -6.95564385000958e-05}, {0.0102054, -7.193072125479842e-05}, {0.0102287, -7.426681544849227e-05}, {0.010252, -7.65653080918821e-05}, {0.010275300000000001, -7.88267780438949e-05}, {0.0102986, -8.1051796094445e-05}, {0.0103219, -8.324092504757994e-05}, {0.0103452, -8.539471980493793e-05}, {0.010368500000000001, -8.751372744945672e-05}, {0.0103918, -8.959848732927114e-05}, {0.0104151, -9.164953114174357e-05}, {0.0104384, -9.366738301757094e-05}, {0.0104617, -9.565255960491938e-05}, {0.010485, -9.760557015353511e-05}, {0.0105083, -9.952691659878713e-05}, {0.0105316, -0.00010141709364559504}, {0.0105549, -0.00010327658885220362}, {0.0105782, -0.00010510588271376186}, {0.0106015, -0.00010690544874567137}, {0.0106248, -0.00010867575356666637}, {0.0106481, -0.00011041725698159475}, {0.010671400000000001, -0.00011213041206386675}, {0.0106947, -0.00011381566523754239}, {0.010718, -0.00011547345635903015}, {0.0107413, -0.00011710421879836908}, {0.010764600000000001, -0.00011870837952007184}, {0.0107879, -0.00012028635916350365}, {0.0108112, -0.00012183857212277698}, {0.0108345, -0.00012336542662613956}, {0.0108578, -0.00012486732481483914}, {0.0108811, -0.00012634466282144527}, {0.0109044, -0.00012779783084761323}, {0.0109277, -0.00012922721324127245}, {0.010951, -0.00013063318857322773}, {0.010974300000000001, -0.00013201612971315826}, {0.0109976, -0.0001333764039050028}, {0.0110209, -0.00013471437284172012}, {0.0110442, -0.00013603039273941302}, {0.011067500000000001, -0.00013732481441080865}, {0.0110908, -0.00013859798333808423}, {0.0111141, -0.00013985023974503249}, {0.0111374, -0.00014108191866855744}, {0.0111607, -0.00014229335002949659}, {0.011184, -0.00014348485870276215}, {0.0112073, -0.00014465676458679742}, {0.0112306, -0.000145809382672343}, {0.0112539, -0.00014694302311051005}, {0.011277200000000001, -0.00014805799128015708}, {0.0113005, -0.00014915458785456735}, {0.0113238, -0.0001502331088674257}, {0.0113471, -0.00015129384577809165}, {0.011370400000000001, -0.00015233708553616943}, {0.0113937, -0.0001533631106453732}, {0.011417, -0.00015437219922668762}, {0.0114403, -0.0001553646250808231}, {0.011463600000000001, -0.00015634065774996792}, {0.0114869, -0.00015730056257883633}, {0.0115102, -0.00015824460077501544}, {0.0115335, -0.00015917302946861077}, {0.0115568, -0.00016008610177119402}, {0.0115801, -0.00016098406683405435}, {0.0116034, -0.0001618671699057558}, {0.0116267, -0.00016273565238900301}, {0.01165, -0.0001635897518968195}, {0.011673300000000001, -0.00016442970230804024}, {0.0116966, -0.000165255733822123}, {0.0117199, -0.00016606807301328157}, {0.0117432, -0.00016686694288394453}, {0.011766500000000001, -0.00016765256291754392}, {0.0117898, -0.00016842514913063792}, {0.0118131, -0.00016918491412437175}, {0.0118364, -0.00016993206713528092}, {0.0118597, -0.00017066681408544213}, {0.011883, -0.00017138935763197607}, {0.0119063, -0.0001720998972159072}, {0.0119296, -0.00017279862911038493}, {0.0119529, -0.00017348574646827226}, {0.011976200000000001, -0.00017416143936910616}, {0.0119995, -0.00017482589486543526}, {0.0120228, -0.0001754792970285404}, {0.0120461, -0.00017612182699354293}, {0.012069400000000001, -0.0001767536630039066}, {0.0120927, -0.00017737498045533866}, {0.012116, -0.00017798595193909558}, {0.0121393, -0.00017858674728469872}, {0.0121626, -0.00017917753360206621}, {0.0121859, -0.00017975847532306655}, {0.0122092, -0.00018032973424249942}, {0.0122325, -0.00018089146955850978}, {0.0122558, -0.0001814438379124409}, {0.012279100000000001, -0.00018198699342813227}]}], 15 "Output Cluster X":T3={"amplitudex"=0.005274459624350753, "temperaturex"=0.0012307264247950805, "alphax"=0.0005350984455630785, "offsetx"=-0.00021373782970607287, "numberx"=132423359.31960036, "peakdensityx"=8593872648510411.0, "centerx"=0.005568390804982347} {"centerx" format="%.2e"; "peakdensityx" format="%.2e"; "numberx" format="%.2e"; "offsetx" format="%.2e"; "alphax" format="%.2e"; "temperaturex" format="%.2e"; "amplitudex" format="%.2e"}, 17 "parameters from\n peak absorption":T5={"abscrosssection"=6.304385518341555e-14, "peakdensity"=1.3847905373010044e+16, "twosizeoneoverezabsxsecdens"=0.9343090057373047, "number"=17767693.746834062} {"number" format="%.2e"; "twosizeoneoverezabsxsecdens" format="%.2e"; "peakdensity" format="%.2e"; "abscrosssection" format="%.2e"}, 18 "Y side":cluster{cluster{dbl, dbl}[]}[](graph)=[{[{0.0, -0.000244320068359375}, {4.63e-05, -0.000281977783203125}, {9.26e-05, -0.00013711219482421874}, {0.00013890000000000002, -0.00032516754150390623}, {0.0001852, -0.0002496103515625}, {0.0002315, -0.0001827309326171875}, {0.00027780000000000003, -0.0002820403564453125}, {0.0003241, -0.00022746511230468751}, {0.0003704, -0.0002171803466796875}, {0.0004167, -0.0001754838134765625}, {0.000463, -0.0003130425537109375}, {0.0005093, -0.0002228346923828125}, {0.0005556000000000001, -0.0001338669189453125}, {0.0006019, -0.0002503896728515625}, {0.0006482, -0.0001243330322265625}, {0.0006945, -0.00021492770996093752}, {0.0007408, -0.000298906689453125}, {0.0007871, -0.0003029056884765625}, {0.0008334, -0.0001866901123046875}, {0.0008797, -0.0003414621826171875}, {0.000926, -0.00044149404296875}, {0.0009723, -0.00022135}, {0.0010186, -0.000207731787109375}, {0.0010649, -0.0003537834228515625}, {0.0011112000000000001, -0.00017838493652343751}, {0.0011575000000000001, -0.0001116818603515625}, {0.0012038, -0.000137695263671875}, {0.0012501, -0.0001945458984375}, {0.0012964, -0.000215900439453125}, {0.0013427, -0.00015345234375}, {0.001389, -0.0002192395751953125}, {0.0014353, -0.00011451472167968751}, {0.0014816, -0.000103063818359375}, {0.0015279, -8.6339697265625e-05}, {0.0015742, -0.00024772177734375}, {0.0016205, -0.0002421982666015625}, {0.0016668, -1.08934326171875e-05}, {0.0017131, -4.2868359375000004e-05}, {0.0017594, -0.0001407044677734375}, {0.0018057, -0.0001495671142578125}, {0.001852, -9.1163525390625e-05}, {0.0018983000000000001, 7.57761962890625e-05}, {0.0019446, -0.000157309130859375}, {0.0019909, -7.602080078125e-05}, {0.0020372, -5.3244140625e-05}, {0.0020835, 1.49436279296875e-05}, {0.0021298, 3.99103515625e-05}, {0.0021761, 3.196923828125e-06}, {0.0022224000000000002, 9.4758642578125e-05}, {0.0022687000000000002, 0.000134259423828125}, {0.0023150000000000002, -7.192509765625e-05}, {0.0023613, 9.95426513671875e-05}, {0.0024076, 0.000113143798828125}, {0.0024539, 0.0001381787841796875}, {0.0025002, 9.55607177734375e-05}, {0.0025465, 3.0001025390625e-05}, {0.0025928, 0.000115350927734375}, {0.0026391, 0.000263865673828125}, {0.0026854, 0.0001266197998046875}, {0.0027317, 8.55489990234375e-05}, {0.002778, 0.0002554751708984375}, {0.0028243, 0.00024557153320312503}, {0.0028706, 0.00022454123535156252}, {0.0029169, 0.00018546708984375}, {0.0029632, 0.0002792814453125}, {0.0030095, 0.0002477502197265625}, {0.0030558, 0.0002661695068359375}, {0.0031021, 0.00023677145996093752}, {0.0031484, 0.0003107557861328125}, {0.0031947, 0.0004321592529296875}, {0.003241, 0.0005389547119140625}, {0.0032873, 0.00047705270996093753}, {0.0033336, 0.0005544614990234375}, {0.0033799, 0.000754371630859375}, {0.0034262, 0.0007216799560546875}, {0.0034725, 0.0006181383056640625}, {0.0035188, 0.00087122431640625}, {0.0035651, 0.0008176445556640625}, {0.0036114, 0.000849448828125}, {0.0036577, 0.001023937158203125}, {0.003704, 0.0008784316162109375}, {0.0037503000000000002, 0.001017645703125}, {0.0037966000000000002, 0.0010463611328125}, {0.0038429000000000002, 0.0012615732666015624}, {0.0038892, 0.0013173089599609375}, {0.0039355, 0.0013993197265625}, {0.0039818, 0.0015721441772460938}, {0.0040281, 0.0015963372680664063}, {0.0040744, 0.0018034546997070314}, {0.0041207, 0.0018722653564453126}, {0.004167, 0.002019741955566406}, {0.0042133, 0.0021332640380859373}, {0.0042596, 0.0023861196655273437}, {0.0043059, 0.0024019506958007815}, {0.0043522, 0.0024828550537109376}, {0.0043985, 0.0024964931762695313}, {0.0044448000000000005, 0.0025025258056640626}, {0.0044911000000000005, 0.0025822242065429686}, {0.0045374000000000005, 0.002668851171875}, {0.0045837000000000004, 0.0028431745361328126}, {0.0046300000000000004, 0.0028808692260742187}, {0.0046763, 0.0029436756958007813}, {0.0047226, 0.003060252490234375}, {0.0047689, 0.0031447263671875}, {0.0048152, 0.003161276989746094}, {0.0048615, 0.0032340183837890626}, {0.0049078, 0.003200305627441406}, {0.0049541, 0.003264500085449219}, {0.0050004, 0.003303397888183594}, {0.0050467, 0.003357927624511719}, {0.005093, 0.003247426123046875}, {0.0051393, 0.003181690087890625}, {0.0051856, 0.003087781872558594}, {0.0052319, 0.0030002248413085937}, {0.0052782, 0.003097500634765625}, {0.0053245, 0.002936516748046875}, {0.0053708, 0.0028459960205078124}, {0.0054171, 0.0026470955932617187}, {0.0054634, 0.00258878017578125}, {0.0055097, 0.0024355269287109375}, {0.005556, 0.00236374404296875}, {0.0056023, 0.0022559900756835938}, {0.0056486, 0.0021902398193359377}, {0.0056949, 0.002039967333984375}, {0.0057412, 0.0019575640625}, {0.0057875, 0.0017610357299804689}, {0.0058338, 0.0015694905029296875}, {0.0058801, 0.001545456689453125}, {0.0059264, 0.0014465511474609375}, {0.0059727, 0.0013871065673828125}, {0.006019, 0.001271112841796875}, {0.0060653, 0.00116870888671875}, {0.0061116, 0.001179482861328125}, {0.0061579, 0.0010268325927734374}, {0.0062042, 0.000960123828125}, {0.0062505, 0.0008706156494140625}, {0.0062968, 0.000830961279296875}, {0.0063431, 0.0007580065673828125}, {0.0063894, 0.0007033744384765626}, {0.0064357, 0.0005814362548828125}, {0.006482, 0.000543715966796875}, {0.0065283, 0.000448331591796875}, {0.0065746, 0.0004073347412109375}, {0.0066209, 0.0003654903076171875}, {0.0066672, 0.00033377705078125}, {0.0067135, 0.000338908056640625}, {0.0067598, 0.00030576699218750003}, {0.0068061, 0.0002659760986328125}, {0.0068524, 0.0001026826904296875}, {0.0068987, 0.000132063671875}, {0.006945, 0.0001647894775390625}, {0.0069913, 4.13267822265625e-05}, {0.0070376, 9.527060546875001e-05}, {0.0070839, 5.94502685546875e-05}, {0.0071302, 9.52990478515625e-05}, {0.0071765, 6.13502197265625e-05}, {0.0072228, -9.240361328125e-05}, {0.0072691, -2.760048828125e-05}, {0.0073154, 2.1968896484375e-05}, {0.0073617, -1.82429443359375e-05}, {0.007408, -7.743154296875e-05}, {0.0074543000000000005, -0.0001287472900390625}, {0.0075006000000000005, -4.1696533203125e-05}, {0.0075469000000000005, -0.00014986291503906252}, {0.0075932000000000005, 4.3767138671875e-05}, {0.0076395000000000005, -4.4091381835937504e-05}, {0.0076858000000000004, -8.24430908203125e-05}, {0.0077321, -2.82660400390625e-05}, {0.0077784, -9.559484863281251e-05}, {0.0078247, -0.0001705007080078125}, {0.007871, -0.00016232636718750001}, {0.0079173, -0.00017222431640625}, {0.0079636, -0.00015270146484375}, {0.0080099, -0.0001376554443359375}, {0.0080562, -0.00016324221191406252}, {0.0081025, -0.00019299863281250002}, {0.0081488, -0.0002751231689453125}, {0.0081951, -9.69600830078125e-05}, {0.0082414, -0.000134145654296875}, {0.0082877, -0.00014146103515625002}, {0.008334, -0.000216526171875}, {0.0083803, -0.00023170871582031251}, {0.0084266, -0.00020999580078125}, {0.0084729, -0.000208118603515625}, {0.0085192, -7.01673583984375e-05}, {0.0085655, -0.0001788627685546875}, {0.0086118, -0.0002609133544921875}, {0.0086581, -0.00023066772460937502}, {0.0087044, -0.000296904345703125}, {0.0087507, -0.000181724072265625}, {0.008797, -0.000108615771484375}, {0.0088433, -0.0002381594482421875}, {0.008889600000000001, -0.0002302240234375}, {0.0089359, -0.0002509016357421875}, {0.008982200000000001, -0.000202873828125}, {0.0090285, -0.00030878757324218753}, {0.009074800000000001, -0.0002097853271484375}, {0.0091211, -0.00024151564941406252}, {0.009167400000000001, -0.0002651740234375}, {0.0092137, -0.0002618690185546875}, {0.009260000000000001, -0.000268370947265625}, {0.0093063, -0.0002885252197265625}, {0.0093526, -0.0003084576416015625}, {0.0093989, -0.0002571134521484375}, {0.0094452, -0.000220041650390625}, {0.0094915, -0.0002020262451171875}, {0.0095378, -0.00021559326171875}, {0.0095841, -0.000280202978515625}, {0.0096304, -0.000189585546875}, {0.0096767, -0.00022018955078125}]}, {[{0.0, -0.00023051806573874898}, {4.63e-05, -0.00023000561610113973}, {9.26e-05, -0.00022945883140248672}, {0.00013890000000000002, -0.00022887542229411232}, {0.0001852, -0.0002282529478924323}, {0.0002315, -0.00022758880586326254}, {0.00027780000000000003, -0.00022688022186959298}, {0.0003241, -0.0002261242383433494}, {0.0003704, -0.00022531770253938054}, {0.0004167, -0.0002244572538275121}, {0.000463, -0.0002235393101760006}, {0.0005093, -0.0002225600537770957}, {0.0005556000000000001, -0.0002215154157626774}, {0.0006019, -0.00022040105995507642}, {0.0006482, -0.0002192123655952081}, {0.0006945, -0.00021794440898705765}, {0.0007408, -0.00021659194399434764}, {0.0007871, -0.00021514938132190058}, {0.0008334, -0.00021361076651078847}, {0.0008797, -0.00021196975657284268}, {0.000926, -0.00021021959518649228}, {0.0009723, -0.0002083530863722207}, {0.0010186, -0.00020636256656219503}, {0.0010649, -0.00020423987497484976}, {0.0011112000000000001, -0.00020197632220142267}, {0.0011575000000000001, -0.00019956265690767496}, {0.0012038, -0.00019698903055031698}, {0.0012501, -0.00019424496000404996}, {0.0012964, -0.00019131928799167333}, {0.0013427, -0.00018820014120646202}, {0.001389, -0.00018487488601305813}, {0.0014353, -0.00018133008161053775}, {0.0014816, -0.000177551430539206}, {0.0015279, -0.00017352372641116323}, {0.0015742, -0.00016923079874391357}, {0.0016205, -0.00016465545477641964}, {0.0016668, -0.00015977941814823636}, {0.0017131, -0.00015458326432490872}, {0.0017594, -0.00014904635265695744}, {0.0018057, -0.0001431467549658087}, {0.001852, -0.00013686118055830662}, {0.0018983000000000001, -0.00013016489758240092}, {0.0019446, -0.0001230316506507073}, {0.0019909, -0.00011543357467646292}, {0.0020372, -0.00010734110488860364}, {0.0020835, -9.872288302003286e-05}, {0.0021298, -8.954565969653112e-05}, {0.0021761, -7.97741930942058e-05}, {0.0022224000000000002, -6.937114398210746e-05}, {0.0022687000000000002, -5.829696732505238e-05}, {0.0023150000000000002, -4.650980069142173e-05}, {0.0023613, -3.3965349793672425e-05}, {0.0024076, -2.0616771587702687e-05}, {0.0024539, -6.4145554736679584e-06}, {0.0025002, 8.693596721648559e-06}, {0.0025465, 2.476289113871927e-05}, {0.0025928, 4.185156162244712e-05}, {0.0026391, 6.002098754542787e-05}, {0.0026854, 7.9335808196797e-05}, {0.0027317, 9.986403190728921e-05}, {0.002778, 0.00012167713771910215}, {0.0028243, 0.00014485016698509765}, {0.0028706, 0.00016946180178547556}, {0.0029169, 0.0001955944264693127}, {0.0029632, 0.00022333416794930984}, {0.0030095, 0.0002527709095845344}, {0.0030558, 0.0002839982725591252}, {0.0031021, 0.0003171135575831761}, {0.0031484, 0.00035221763848042504}, {0.0031947, 0.0003894147977574319}, {0.003241, 0.00042881249253821213}, {0.0032873, 0.0004705210372602679}, {0.0033336, 0.0005146531872219027}, {0.0033799, 0.0005613236044019663}, {0.0034262, 0.0006106481838938367}, {0.0034725, 0.0006627432157557333}, {0.0035188, 0.0007177243530302183}, {0.0035651, 0.0007757053520825287}, {0.0036114, 0.0008367965462169012}, {0.0036577, 0.0009011030077399987}, {0.003704, 0.0009687223472743979}, {0.0037503000000000002, 0.0010397420922636609}, {0.0037966000000000002, 0.0011142365794231588}, {0.0038429000000000002, 0.0011922632886797392}, {0.0038892, 0.0012738585394051903}, {0.0039355, 0.0013590324642592591}, {0.0039818, 0.0014477631728859906}, {0.0040281, 0.0015399900187606996}, {0.0040744, 0.001635605890096582}, {0.0041207, 0.0017344484632642097}, {0.004167, 0.001836290389203131}, {0.0042133, 0.0019408284357396324}, {0.0042596, 0.0020476716889573873}, {0.0043059, 0.0021563290334485384}, {0.0043522, 0.0022661962935548122}, {0.0043985, 0.002376543633510798}, {0.0044448000000000005, 0.002486504087111287}, {0.0044911000000000005, 0.0025950644104251815}, {0.0045374000000000005, 0.0027010597988173833}, {0.0045837000000000004, 0.002803174326238401}, {0.0046300000000000004, 0.0028999491488821507}, {0.0046763, 0.002989800401326928}, {0.0047226, 0.0030710480443405463}, {0.0047689, 0.0031419552816516743}, {0.0048152, 0.0032007746921724387}, {0.0048615, 0.0032457893022505547}, {0.0049078, 0.003275311825954257}, {0.0049541, 0.0032874356774864944}, {0.0050004, 0.0032791738865833864}, {0.0050467, 0.0032529309753080806}, {0.005093, 0.003210854985713626}, {0.0051393, 0.0031546388013195853}, {0.0051856, 0.0030859908283279837}, {0.0052319, 0.0030066551857468975}, {0.0052782, 0.0029183745282829556}, {0.0053245, 0.0028228435864997353}, {0.0053708, 0.002721667952145628}, {0.0054171, 0.0026163330274581475}, {0.0054634, 0.002508184022001144}, {0.0055097, 0.0023984159684184336}, {0.005556, 0.0022880719073225227}, {0.0056023, 0.0021780471915042073}, {0.0056486, 0.00206909800022598}, {0.0056949, 0.001961852454584041}, {0.0057412, 0.001856823072162567}, {0.0057875, 0.001754419629825035}, {0.0058338, 0.0016549617871361552}, {0.0058801, 0.001558691049953605}, {0.0059264, 0.0014657818260820719}, {0.0059727, 0.001376351449887023}, {0.006019, 0.0012904691395088047}, {0.0060653, 0.0012081639076335056}, {0.0061116, 0.0011294314823335956}, {0.0061579, 0.0010542403145052213}, {0.0062042, 0.0009825367577086547}, {0.0062505, 0.0009142495083527605}, {0.0062968, 0.0008492933917547523}, {0.0063431, 0.0007875725744890675}, {0.0063894, 0.0007289832768764702}, {0.0064357, 0.0006734160523002372}, {0.006482, 0.0006207576928150233}, {0.0065283, 0.0005708928135709719}, {0.0065746, 0.0005237051621025141}, {0.0066209, 0.00047907869262365057}, {0.0066672, 0.000436898440162189}, {0.0067135, 0.0003970512246478518}, {0.0067598, 0.0003594262109133369}, {0.0068061, 0.0003239153469304638}, {0.0068524, 0.00029041369943685734}, {0.0068987, 0.0002588197033623325}, {0.006945, 0.0002290353390898135}, {0.0069913, 0.00020096624953787868}, {0.0070376, 0.00017452180728933894}, {0.0070839, 0.00014961514047526109}, {0.0071302, 0.00012616312482331476}, {0.0071765, 0.00010408634816399101}, {0.0072228, 8.33090527325065e-05}, {0.0072691, 6.375905978579822e-05}, {0.0073154, 4.53676803536144e-05}, {0.0073617, 2.806961534364163e-05}, {0.007408, 1.1802847708492655e-05}, {0.0074543000000000005, -3.491471055158194e-06}, {0.0075006000000000005, -1.7869138178594697e-05}, {0.0075469000000000005, -3.13830190863162e-05}, {0.0075932000000000005, -4.408316774839348e-05}, {0.0076395000000000005, -5.6016946845311175e-05}, {0.0076858000000000004, -6.722914686768482e-05}, {0.0077321, -7.776210344067267e-05}, {0.0077784, -8.765581230498948e-05}, {0.0078247, -9.694804150680265e-05}, {0.007871, -0.0001056744404505615}, {0.0079173, -0.00011386864555465051}, {0.0079636, -0.00012156238232194855}, {0.0080099, -0.00012878556369790573}, {0.0080562, -0.00013556638463926426}, {0.0081025, -0.00014193141285855795}, {0.0081488, -0.0001479056757442003}, {0.0081951, -0.00015351274348445504}, {0.0082414, -0.00015877480844672526}, {0.0082877, -0.00016371276088224962}, {0.008334, -0.0001683462610410769}, {0.0083803, -0.0001726938077937398}, {0.0084266, -0.00017677280386481435}, {0.0084729, -0.00018059961779001151}, {0.0085192, -0.00018418964271292484}, {0.0085655, -0.00018755735214041278}, {0.0086118, -0.00019071635277705763}, {0.0086581, -0.00019367943455948528}, {0.0087044, -0.00019645861801071573}, {0.0087507, -0.0001990651990333459}, {0.008797, -0.00020150979125836037}, {0.0088433, -0.0002038023660638739}, {0.008889600000000001, -0.00020595229037521112}, {0.0089359, -0.00020796836235453898}, {0.008982200000000001, -0.00020985884508484062}, {0.0090285, -0.0002116314983494349}, {0.009074800000000001, -0.0002132936086045524}, {0.0091211, -0.00021485201723871788}, {0.009167400000000001, -0.00021631314720890993}, {0.0092137, -0.0002176830281396875}, {0.009260000000000001, -0.00021896731996773292}, {0.0093063, -0.00022017133521056475}, {0.0093526, -0.00022130005993455812}, {0.0093989, -0.00022235817349386977}, {0.0094452, -0.00022335006710842603}, {0.0094915, -0.000224279861345792}, {0.0095378, -0.00022515142256851196}, {0.0095841, -0.0002259683784053938}, {0.0096304, -0.00022673413230221202}, {0.0096767, -0.00022745187720441863}]}], 19 "Output ClusterY":T2={"amplitudey"=0.009583848983012275, "temperaturey"=0.00128830129384577, "alphay"=0.0005601309973242479, "offsety"=-0.0002381406803704182, "numbery"=125936758.9561993, "peakdensityy"=7125397095110792.0, "centery"=0.004958691987542826} {"centery" format="%.2e"; "peakdensityy" format="%.2e"; "numbery" format="%.2e"; "offsety" format="%.2e"; "alphay" format="%.2e"; "temperaturey" format="%.2e"; "amplitudey" format="%.2e"})   [LabVIEW 2013]
uses:
  <vilib>/Utility/file.llb/Read From Spreadsheet File (DBL).vi
panel:
  in  "number of rows (all:-1)":i32=-1
  out "alpha guess 2":dbl=10.448588597444687 format="%.2e"
  in  "model description Y":T4={"model"="a*exp(-((1+(abs((y-c))/(1.256*b))^1.9086))^(1/1.9086))+d", "Parameters"=["a", "b", "c", "d"], "x"="y"}
  in  "model description X":T4={"model"="a*exp(-((1+(abs((x-c)/2)/(1.256*b))^1.9086))^(1/1.9086))+d", "Parameters"=["a", "b", "c", "d"], "x"="x"}
  out "bckgrnd peak value\nminus camera bckgrnd":sgl=56.0 format="%.2f"
  out "atom peak value\nminus camera bckgrnd":sgl=22.0 format="%.2f"
  out "bckgrnd Pixel Value":sgl=71.0 format="%.2f"
  out "atom Pixel Value":sgl=37.0 format="%.2f"
  out "bgrnd and\natom image\n same size?":bool=TRUE
  in  "File Path for \natom image":path=path "C:/data/MOT/08.05.02/metapic600c1.0v40aa.bmp"
  # "see page 68  of sr lab notebook #1"
  # "(old info)"
  # "y-axis  is strong field gradient"
  # "(8/02)"
  # "edit help/manually call file\nfor editing"
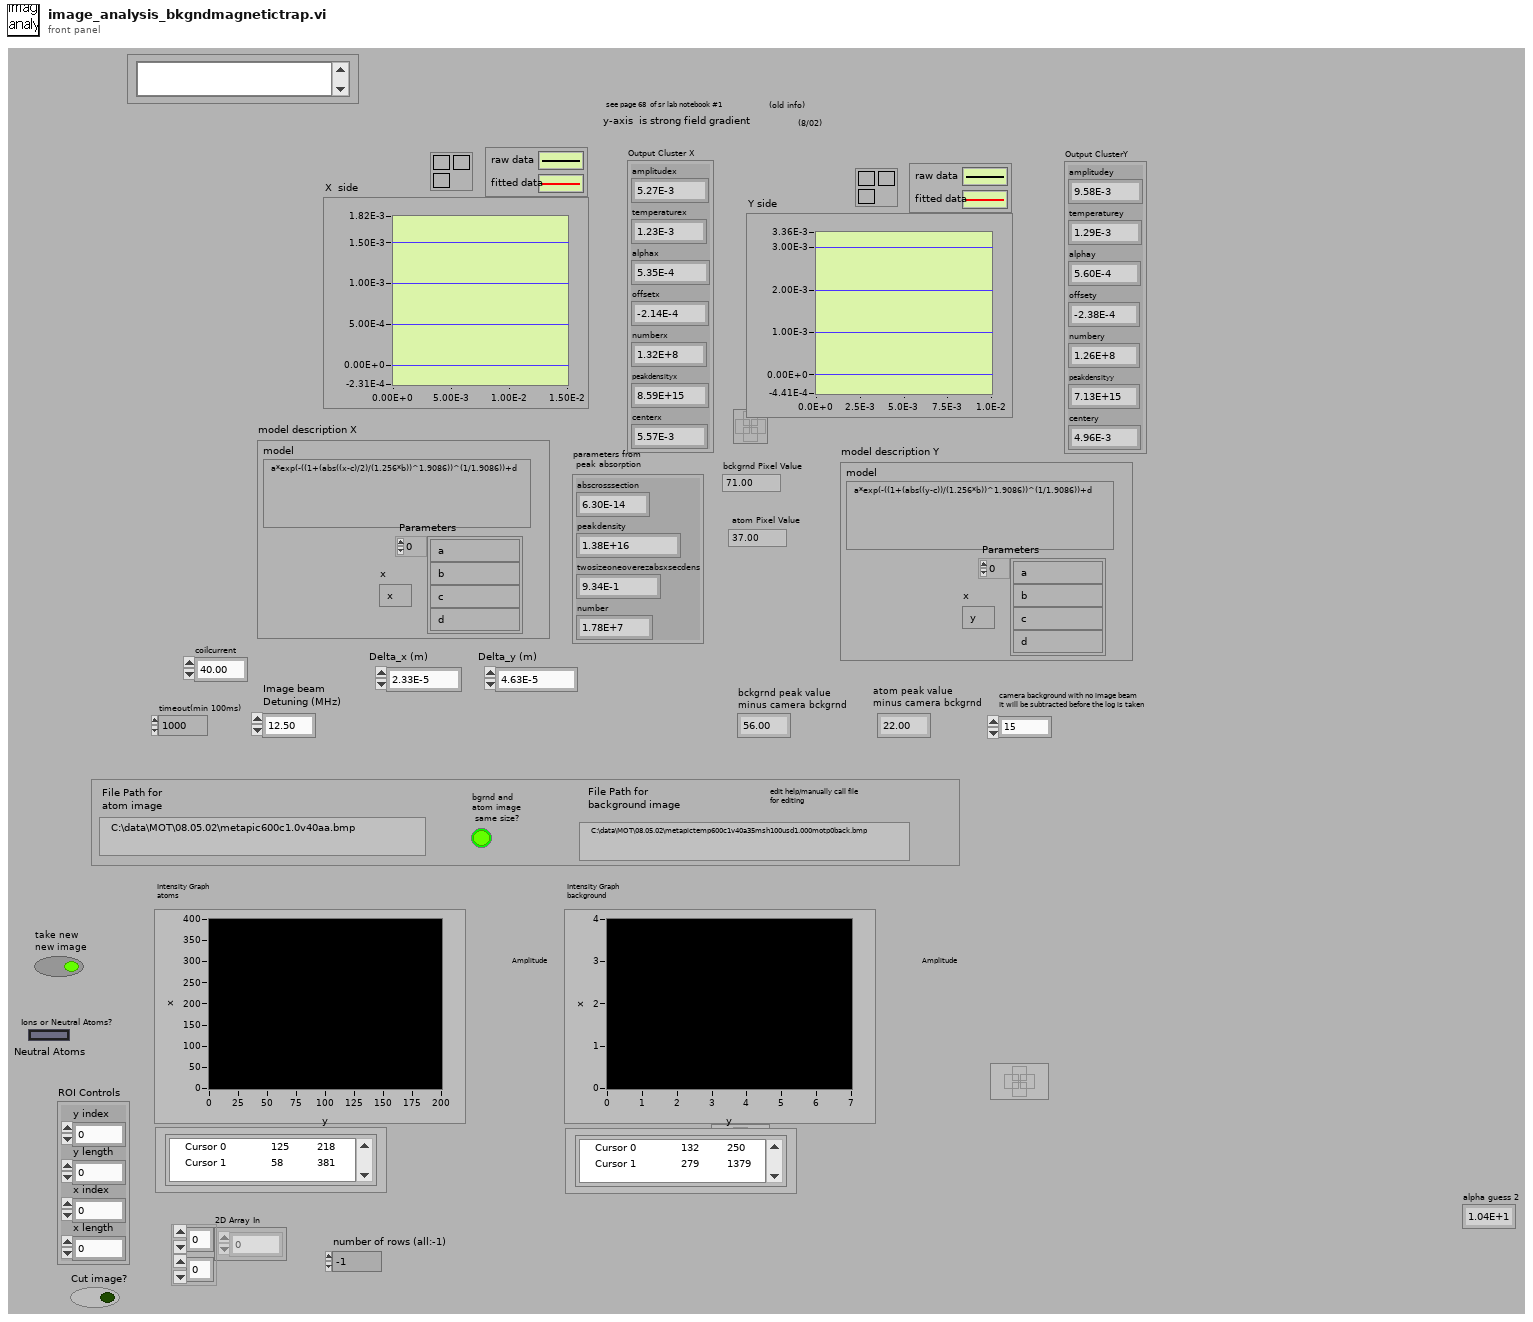
[diagram p1: front panel]
types:
  T1 = cluster{"y index":i32, "y length":i32, "x index":i32, "x length":i32}
  T2 = cluster{"amplitudey":dbl, "temperaturey":dbl, "alphay":dbl, "offsety":dbl, "numbery":dbl, "peakdensityy":dbl, "centery":dbl}
  T3 = cluster{"amplitudex":dbl, "temperaturex":dbl, "alphax":dbl, "offsetx":dbl, "numberx":dbl, "peakdensityx":dbl, "centerx":dbl}
  T4 = cluster{"model":string, "Parameters":string[], "x":string}
  T5 = cluster{"abscrosssection":dbl, "peakdensity":dbl, "twosizeoneoverezabsxsecdens":dbl, "number":dbl}
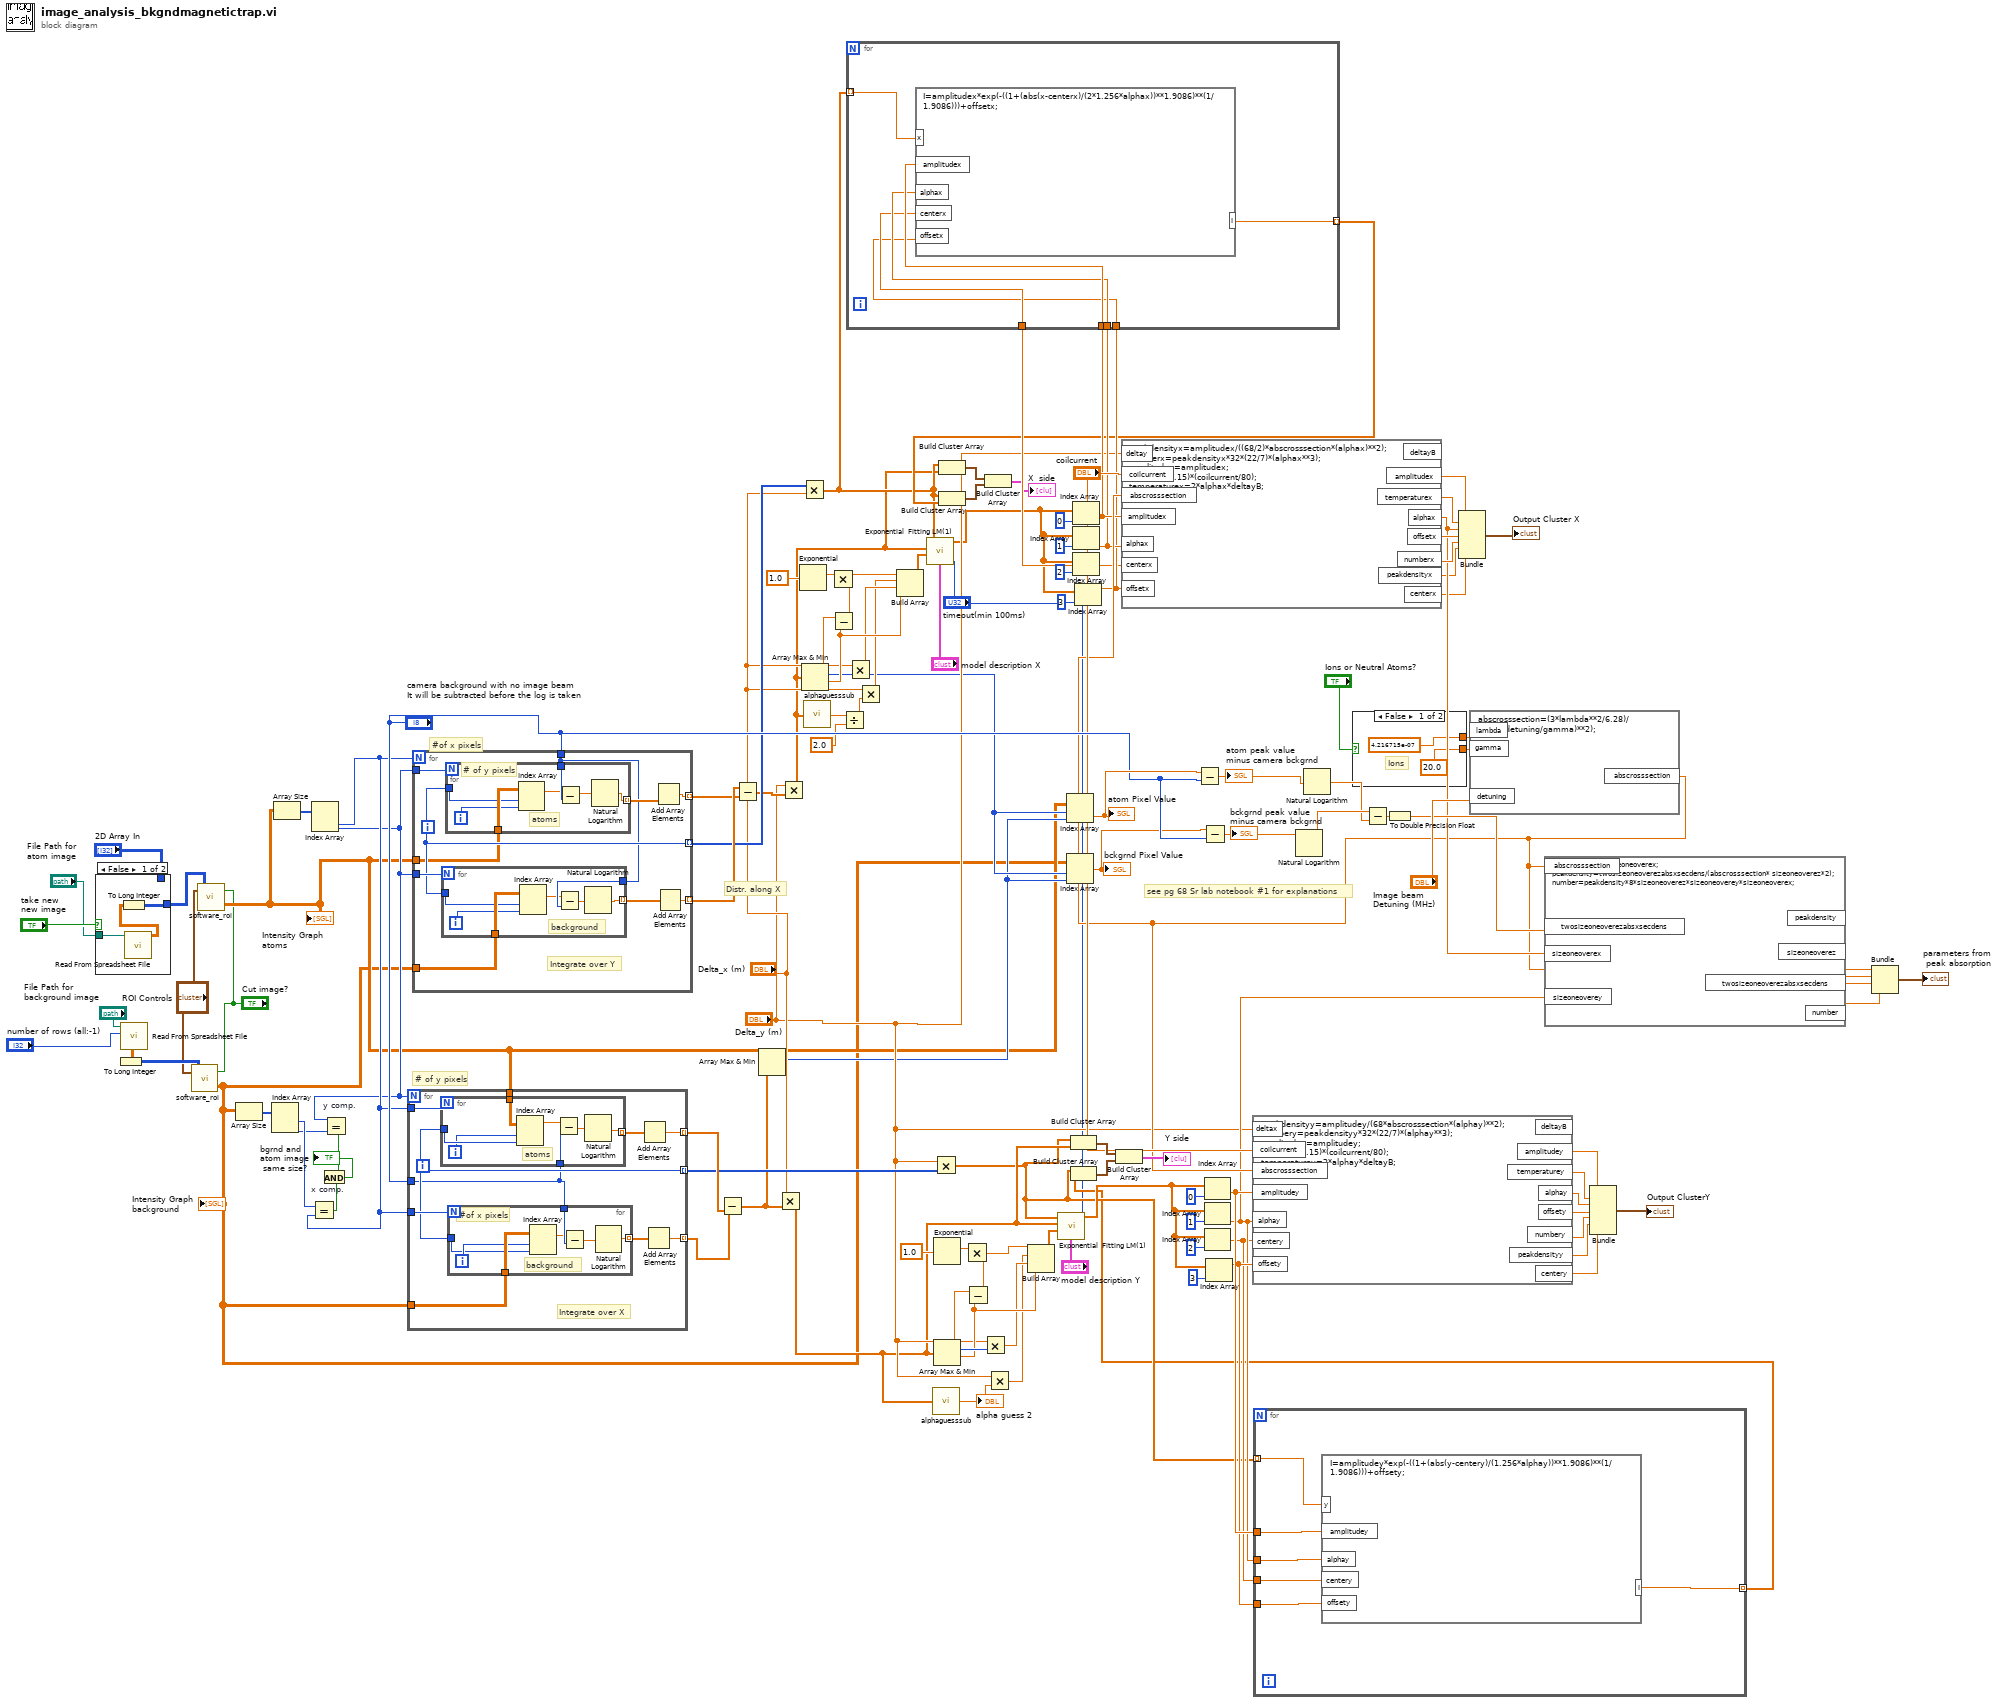
[diagram p0: block diagram]
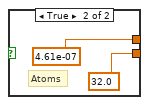
[diagram p2: hidden frame]
diagram:
  # "#of x pixels"
  # "data fromabs at center"
  # "see pg 68 Sr lab notebook #1 for explanations"
  # "# of y pixels"
  # "Distr. along X"
  n1 = case shown="False" "take new\nnew image" {
    tunnel: [w127 w128] -> w5
    tunnel: "2D Array In" -> [_ w128]
    tunnel: "File Path for \natom image" -> [w125 _]
    frame False {
      n2 = call-poly <vilib>:"Read From Spreadsheet File.vi"("file path (dialog if empty)"=w125) -> ("all rows"=w126:dbl[][])  [unwired: 6 in, 4 out]
      n3 = To Long Integer(number=w126) -> (32bit integer=w127:i32[][])
    }
    frame True {
    }
  }
  n4 = call-poly <vilib>:"Read From Spreadsheet File.vi"("number of rows (all:-1)"="number of rows (all:-1)", "file path (dialog if empty)"="File Path for \nbackground image") -> ("all rows"=w19:dbl[][])  [unwired: 5 in, 4 out]
  n5 = To Long Integer(number=w19) -> (32bit integer=w3:i32[][])
  n6 = call "software_roi.vi"("Cut image?"="Cut image?", "Input Array"=w3, "ROI Controls"="ROI Controls") -> ("output array"=w4:sgl[][])
  "Intensity Graph \nbackground" <- w4
  n7 = call "software_roi.vi"("Cut image?"="Cut image?", "Input Array"=w5, "ROI Controls"="ROI Controls") -> ("output array"=w6:sgl[][])
  "Intensity Graph \natoms" <- w6
  n8 = Array Size(array=w4) -> (size(s)=w17:i32[])
  n9 = Index Array(array=w17) -> (element #1=w16:i32, element #2=w15:i32)  [unwired: 2 in]
  n10 = Array Size(array=w6) -> (size(s)=w12:i32[])
  n11 = Index Array(array=w12) -> (element #1=w11:i32, element #2=w10:i32)  [unwired: 2 in]
  n12 = Equal? "x comp."(x=w16, y=w11) -> (x = y?=w119:bool)
  n13 = Equal? "y comp."(x=w10, y=w15) -> (x = y?=w120:bool)
  n14 = And(x=w120, y=w119) -> (x .and. y?=→"bgrnd and\natom image\n same size?":bool)
  n15 = for {
    N: w10 -> [_]
    tunnel: w11 -> [w138]
    tunnel: [w136] -> w123 mode=indexing
    tunnel: w11 -> [w135]
    tunnel: [w133] -> w124 mode=indexing
    tunnel: [w132] -> w69 mode=indexing
    tunnel: "camera background with no image beam\nIt will be subtracted before the log is taken" -> [w131]
    tunnel: w4 -> [w130]
    tunnel: w6 -> [w129]
    i -> [w132]
    # "Integrate over X"
    n16 = for {
      N: w138 -> [_]
      tunnel: [w152] -> w137 mode=indexing
      tunnel: w132 -> [w147]
      tunnel: w131 -> [w150]
      tunnel: w129 -> [w149]
      i -> [w146]
      # "atoms"
      n17 = Index Array(array=w149, index (row)=w146, index (col)=w147) -> (element=w148:sgl)
      n18 = Subtract(x=w148, y=w150) -> (x-y=w151:sgl)
      n19 = Natural Logarithm(1:w151) -> (0:w152:sgl)
    }
    n20 = for {
      N: w135 -> [_]
      tunnel: [w145] -> w134 mode=indexing
      tunnel: w130 -> [w142]
      tunnel: w132 -> [w139]
      tunnel: w131 -> [w143]
      i -> [w140]
      # "background"
      # "#of x pixels"
      n21 = Index Array(array=w142, index (row)=w140, index (col)=w139) -> (element=w141:sgl)
      n22 = Subtract(x=w141, y=w143) -> (x-y=w144:sgl)
      n23 = Natural Logarithm(1:w144) -> (0:w145:sgl)
    }
    n24 = Add Array Elements(numeric array=w137) -> (sum=w136:sgl)
    n25 = Add Array Elements(numeric array=w134) -> (sum=w133:sgl)
  }
  n26 = for {
    N: w11 -> [_]
    tunnel: w10 -> [w162]
    tunnel: [w160] -> w121 mode=indexing
    tunnel: w10 -> [w159]
    tunnel: [w157] -> w122 mode=indexing
    tunnel: [w156] -> w92 mode=indexing
    tunnel: "camera background with no image beam\nIt will be subtracted before the log is taken" -> [w155]
    tunnel: w4 -> [w154]
    tunnel: w6 -> [w153]
    i -> [w156]
    # "Integrate over Y"
    n27 = for {
      N: w159 -> [_]
      tunnel: w156 -> [w164]
      tunnel: [w169] -> w158 mode=indexing
      tunnel: w155 -> [w167]
      tunnel: w154 -> [w166]
      i -> [w165]
      # "background"
      n28 = Index Array(array=w166, index (row)=w164, index (col)=w165) -> (element=w163:sgl)
      n29 = Subtract(x=w163, y=w167) -> (x-y=w168:sgl)
      n30 = Natural Logarithm(1:w168) -> (0:w169:sgl)
    }
    n31 = for {
      N: w162 -> [_]
      tunnel: w156 -> [w170]
      tunnel: [w176] -> w161 mode=indexing
      tunnel: w155 -> [w174]
      tunnel: w153 -> [w173]
      i -> [w171]
      # "# of y pixels"
      # "atoms"
      n32 = Index Array(array=w173, index (row)=w170, index (col)=w171) -> (element=w172:sgl)
      n33 = Subtract(x=w172, y=w174) -> (x-y=w175:sgl)
      n34 = Natural Logarithm(1:w175) -> (0:w176:sgl)
    }
    n35 = Add Array Elements(numeric array=w161) -> (sum=w160:sgl)
    n36 = Add Array Elements(numeric array=w158) -> (sum=w157:sgl)
  }
  n37 = Subtract(x=w124, y=w123) -> (x-y=w56:sgl[])
  n38 = Subtract(x=w122, y=w121) -> (x-y=w57:sgl[])
  n39 = Array Max & Min(array=w56) -> (max index (indices)=w13:i32)  [unwired: 3 out]
  n40 = Multiply(x="Delta_x (m)", y=w56) -> (x*y=w27:dbl[])
  n41 = Multiply(x="Delta_y (m)", y=w57) -> (x*y=w23:dbl[])
  n42 = Exponential(1:1.0 ("x")) -> (0:w67:dbl)
  n43 = Multiply(x=w92, y="Delta_x (m)") -> (x*y=w24:dbl[])
  n44 = Array Max & Min(array=w23) -> (max value=w65:dbl, max index (indices)=w14:i32, min value=w45:dbl)  [unwired: 1 out]
  n45 = call "alphaguesssub.vi"("Input array"=w23) -> ("alpha guess"=w34:dbl)
  n46 = Subtract(x=w65, y=w45) -> (x-y=w64:dbl)
  n47 = Multiply(x=w67, y=w64) -> (x*y=w68:dbl)
  n48 = Divide(x=w34, y=2.0) -> (x/y=w33:dbl)
  n49 = Multiply(x="Delta_x (m)", y=w14) -> (x*y=w44:dbl)
  n50 = Multiply(x="Delta_x (m)", y=w33) -> (x*y=w38:dbl)
  n51 = Build Array(w68, w38, w44, w45) -> (w93:dbl[])
  n52 = call "Exponential  Fitting LM(1).vi"("X Values"=w24, "Y Values"=w23, "Initial Guess Coefficient"=w93, "model description"="model description X", "timeout(min 100ms)"="timeout(min 100ms)") -> ("Coefficients"=w30:dbl[])  [unwired: 2 in, 1 out]
  n53 = Multiply(x="Delta_y (m)", y=w69) -> (x*y=w26:dbl[])
  n54 = call "alphaguesssub.vi"("Input array"=w27) -> ("alpha guess"=w37:dbl)
  "alpha guess 2" <- w37
  n55 = Exponential(1:1.0 ("x")) -> (0:w63:dbl)
  n56 = Array Max & Min(array=w27) -> (max value=w60:dbl, max index (indices)=w74:i32, min value=w42:dbl)  [unwired: 1 out]
  n57 = Build Cluster Array(w24, w23) -> (w103:cluster{dbl, dbl}[])
  n58 = Subtract(x=w60, y=w42) -> (x-y=w61:dbl)
  n59 = Multiply(x=w63, y=w61) -> (x*y=w59:dbl)
  n60 = Multiply(x="Delta_y (m)", y=w74) -> (x*y=w41:dbl)
  n61 = Multiply(x="Delta_y (m)", y=w37) -> (x*y=w35:dbl)
  n62 = Build Array(w59, w35, w41, w42) -> (w79:dbl[])
  n63 = call "Exponential  Fitting LM(1).vi"("X Values"=w26, "Y Values"=w27, "Initial Guess Coefficient"=w79, "model description"="model description Y", "timeout(min 100ms)"="timeout(min 100ms)") -> ("Coefficients"=w77:dbl[])  [unwired: 2 in, 1 out]
  n64 = Index Array(array=w6, index (row)=w14, index (col)=w13) -> (element=w117:sgl)
  "atom Pixel Value" <- w117
  n65 = Index Array(array=w4, index (row)=w14, index (col)=w13) -> (element=w18:sgl)
  "bckgrnd Pixel Value" <- w18
  n66 = Build Cluster Array(w26, w27) -> (w89:cluster{dbl, dbl}[])
  n67 = Index Array(array=w30, index=0 ("Index")) -> (element=w52:dbl)
  n68 = Index Array(array=w30, index=1 ("Index")) -> (element=w51:dbl)
  n69 = Index Array(array=w30, index=2 ("Index")) -> (element=w43:dbl)
  n70 = Index Array(array=w30, index=3 ("Index")) -> (element=w50:dbl)
  n71 = for {
    tunnel: w24 -> [w182] mode=indexing
    tunnel: w52 -> [w181]
    tunnel: w51 -> [w180]
    tunnel: w43 -> [w179]
    tunnel: w50 -> [w178]
    tunnel: [w177] -> w28 mode=indexing
    n72 = formula code="I=amplitudex*exp(-((1+(abs(x-centerx)/(2*1.256*alphax))**1.9086)**(1/1.9086)))+offsetx;"("amplitudex"=w181, "alphax"=w180, "centerx"=w179, "offsetx"=w178, "x"=w182) -> ("I"=w177:dbl)
  }
  n73 = Build Cluster Array(w24, w28) -> (w29:cluster{dbl, "I":dbl}[])
  n74 = Build Cluster Array(w103, w29) -> (→"X  side":cluster{cluster{dbl, "I":dbl}[]}[])
  n75 = Subtract(x=w117, y="camera background with no image beam\nIt will be subtracted before the log is taken") -> (x-y=w116:sgl)
  "atom peak value\nminus camera bckgrnd" <- w116
  n76 = Subtract(x=w18, y="camera background with no image beam\nIt will be subtracted before the log is taken") -> (x-y=w115:sgl)
  "bckgrnd peak value\nminus camera bckgrnd" <- w115
  n77 = Index Array(array=w77, index=0 ("Index")) -> (element=w49:dbl)
  n78 = Index Array(array=w77, index=1 ("Index")) -> (element=w46:dbl)
  n79 = Index Array(array=w77, index=2 ("Index")) -> (element=w40:dbl)
  n80 = Index Array(array=w77, index=3 ("Index")) -> (element=w48:dbl)
  n81 = for {
    tunnel: w26 -> [w188] mode=indexing
    tunnel: [w187] -> w25 mode=indexing
    tunnel: w49 -> [w186]
    tunnel: w46 -> [w185]
    tunnel: w40 -> [w184]
    tunnel: w48 -> [w183]
    n82 = formula code="I=amplitudey*exp(-((1+(abs(y-centery)/(1.256*alphay))**1.9086)**(1/1.9086)))+offsety;"("amplitudey"=w186, "alphay"=w185, "centery"=w184, "offsety"=w183, "y"=w188) -> ("I"=w187:dbl)
  }
  n83 = Build Cluster Array(w26, w25) -> (w88:cluster{dbl, "I":dbl}[])
  n84 = Build Cluster Array(w89, w88) -> (→"Y side":cluster{cluster{dbl, "I":dbl}[]}[])
  n85 = Natural Logarithm(1:w115) -> (0:w114:sgl)
  n86 = Natural Logarithm(1:w116) -> (0:w113:sgl)
  n87 = case shown="False" "Ions or Neutral Atoms?" {
    tunnel: [20.0 ("Input Variable") 32.0 ("Input Variable")] -> w111
    tunnel: [4.216715e-07 ("Input Variable") 4.61e-07 ("Input Variable")] -> w110
    frame False {
      # "Ions"
    }
    frame True {
      # "Atoms"
    }
  }
  n88 = Subtract(x=w114, y=w113) -> (x-y=w108:sgl)
  n89 = To Double Precision Float(number=w108) -> (double precision float=w105:dbl)
  n90 = formula code="abscrosssection=(3*lambda**2/6.28)/(1+(2*detuning/gamma)**2);"("lambda"=w110, "gamma"=w111, "detuning"="Image beam \nDetuning (MHz)") -> ("abscrosssection"=w58:dbl)
  n91 = formula code="peakdensityx=amplitudex/((68/2)*abscrosssection*(alphax)**2);\nnumberx=peakdensityx*32*(22/7)*(alphax**3);\namplitudex=amplitudex;\ndeltayB=(1.15)*(coilcurrent/80);\ntemperaturex=2*alphax*deltayB;"("amplitudex"=w52, "alphax"=w51, "centerx"=w43, "abscrosssection"=w58, "deltay"="Delta_y (m)", "coilcurrent"="coilcurrent", "offsetx"=w50) -> ("numberx"=w97:dbl, "alphax"=w72:dbl, "offsetx"=w98:dbl, "amplitudex"=w99:dbl, "temperaturex"=w95:dbl, "peakdensityx"=w54:dbl, "centerx"=w53:dbl)  [unwired: 1 out]
  n92 = formula code="peakdensityy=amplitudey/(68*abscrosssection*(alphay)**2);\nnumbery=peakdensityy*32*(22/7)*(alphay**3);\namplitudey=amplitudey;\ndeltayB=(1.15)*(coilcurrent/80);\ntemperaturey=2*alphay*deltayB;"("amplitudey"=w49, "alphay"=w46, "centery"=w40, "abscrosssection"=w58, "deltax"="Delta_y (m)", "coilcurrent"="coilcurrent", "offsety"=w48) -> ("numbery"=w81:dbl, "alphay"=w83:dbl, "offsety"=w82:dbl, "amplitudey"=w84:dbl, "temperaturey"=w80:dbl, "peakdensityy"=w75:dbl, "centery"=w71:dbl)  [unwired: 1 out]
  n93 = Bundle("amplitudex"=w99, "temperaturex"=w95, "alphax"=w72, "offsetx"=w98, "numberx"=w97, "peakdensityx"=w54, "centerx"=w53) -> (→"Output Cluster X":T3)  [unwired: 1 in]
  n94 = formula code="sizeoneoverez=sizeoneoverex;\npeakdensity=twosizeoneoverezabsxsecdens/(abscrosssection* sizeoneoverez*2);\nnumber=peakdensity*8*sizeoneoverez*sizeoneoverey*sizeoneoverex;"("abscrosssection"=w58, "twosizeoneoverezabsxsecdens"=w105, "sizeoneoverex"=w72, "sizeoneoverey"=w46) -> ("peakdensity"=w109:dbl, "twosizeoneoverezabsxsecdens"=w107:dbl, "number"=w106:dbl)  [unwired: 1 out]
  n95 = Bundle("amplitudey"=w84, "temperaturey"=w80, "alphay"=w83, "offsety"=w82, "numbery"=w81, "peakdensityy"=w75, "centery"=w71) -> (→"Output ClusterY":T2)  [unwired: 1 in]
  n96 = Bundle("abscrosssection"=w58, "peakdensity"=w109, "twosizeoneoverezabsxsecdens"=w107, "number"=w106) -> (→"parameters from\n peak absorption":T5)  [unwired: 1 in]
